vi "VP_NanoPositioner_FPGA_diagonal.vi"() -> ()   [LabVIEW 2015]
uses:
  FPGA states.ctl
  FPGA Commands.ctl
  <vilib>/Platform/TimedLoop/XDataNode/timing_clust.ctl
  <vilib>/Platform/TimedLoop/XDataNode/nitl_modes.ctl
  <vilib>/Platform/TimedLoop/XDataNode/wakeup.ctl
  Control X Up Down Ramp.ctl
  Control Y Up Down Ramp.ctl
  Detector_Trigger_Control.ctl
  <vilib>/rvi/Emulation/niFpgaGetClockAttributes.vi
  <vilib>/rvi/Emulation/niFpgaSctlEmulationGetInTimedLoop.vi
  <vilib>/rvi/Emulation/niFpgaEmulationReportErrorSimple.vi
  <vilib>/rvi/eio/common/nirviEmuTemplateMethod_errors.vi
  <vilib>/rvi/Emulation/niFpgaCriticalErrorInLSC.vi
  <vilib>/rvi/Emulation/niFpgaProcessEmulError.vi
  <vilib>/rvi/interface/RandomDataEmulation/niFpgaRandomDataHandleErrors.vi
  <vilib>/eio/EIONode/EIONode.xnode
  <vilib>/Platform/TimedLoop/XDataNode/XDataNode.xnode
  <vilib>/rvi/DataTransferAndStorage/Container/XNode/niFpgaContainer.xnode
  <vilib>/rvi/interface/RandomDataEmulation/nirviRandomDataFpgaReadWriteTemplate.vi
  <vilib>/rvi/Analysis/measure/butterworth/XNode/niFpgaButterworthFilter.xnode
  <vilib>/Platform/TimedLoop/XDataNode/XDNodeRunTimeDep.lvlib
panel:
  out "Interferometer Loop Error":errorcluster
  out "Fly scan completed":bool
  out "Y scan done":bool=TRUE
  out "X scan done":bool=TRUE
  out "Wait error":errorcluster
  out "Shutdown error":errorcluster
  out "FPGA error monitor":errorcluster
  out "Run Loop error":errorcluster
  in  "Wait timer (ms)":u16=50 caption="Count(mSec)"
  in  "New FPGA command":bool
  in  "FPGA command":T1
  out "FPGA state":T2
  out "End Run Error":errorcluster
  out "Number of Data Strings 2":i32
  out "Measured Data Trigger Time Period (Ticks)":u32
  in  "Data Trigger Time Period (uSec)":u32 caption="Detector Trigger Time Period (uSec)"
  out "Trigger for Data":fxp<+/-,58,25>
  out "Fly Scan Running":bool
  in  "Fly Scan":bool
  out "If True End Y Down Ramp":bool
  in  "Y Ramp Drop Size (nm)":fxp<+/-,16,16>
  out "Ramp Mid Range":bool
  out "If True End Up Ramp":bool
  out "Start or middle":bool=TRUE
  in  "Y Start Marker (nm)":fxp<+/-,58,25> format="%#_55g"
  out "Y Ramp Slope":fxp<+,48,16>
  in  "Y Ramp End (nm)":fxp<+/-,16,16>
  in  "Y Ramp Start (nm)":fxp<+/-,16,16>
  in  "Y Ramp Period (usec)":fxp<+,32,32>
  in  "X Ramp Period (usec)":fxp<+,32,32>
  in  "X Ramp End (nm)":fxp<+/-,16,16>
  in  "X Ramp Start (nm)":fxp<+/-,16,16>
  out "If True End X Down Ramp":bool
  out "X Ramp Mid Range":bool
  out "If True End X Up Ramp":bool
  out "Y Ramp Drop":bool
  out "Next Do Down Ramp":bool
  out "Continue Run":bool
  in  "X Start Marker (nm)":fxp<+/-,58,25>
  out "X Ramp Slope":fxp<+,48,16> format="%.37g"
  in  "DT Reset":bool
  in  "DT Duty Cycle (periods)":fxp<+,32,0>=0.5 caption="DT duty cycle (periods)"
  in  "DT Reference DC Offset (V)":fxp<+/-,16,16>
  in  "DT Reference Amplitude (V)":fxp<+/-,40,17>
  in  "DT Phase Offset (periods)":fxp<+,32,0>
  in  "DT Frequency (periods/tick)":fxp<+,32,0>=0.0002500000409781933
  in  "Trigger Wave Generator":T3(ring)
  out "If True End Trigger Low":bool
  in  "Trigger Low Level (V)":fxp<+/-,20,5>=-5.0
  in  "Trigger High Level (V)":fxp<+/-,20,5>=5.0
  out "If True End Trigger High":bool
  out "Trigger Mid High":bool
  in  "Trigger Low Period (usec)":fxp<+/-,64,45>
  in  "Trigger High Period (usec)":fxp<+/-,64,45>
  out "Measured Z Reference Time Period (Ticks)":u32
  in  "Z Reference Time Period (uSec)":u32
  in  "Z White Noise Amplitude":u16=32767
  in  "Z White Noise Seed":u32=4
  in  "Z Phase Offset (periods)":fxp<+,32,0>
  in  "Z Frequency (periods/tick)":fxp<+,32,0>=0.0002500000409781933
  in  "Z Reference DC Offset (nm)":fxp<+/-,16,16>
  in  "Z Reference Amplitude (nm)":fxp<+/-,40,17>
  in  "Z Reference Reset":bool
  in  "Z Reference Wave Selection":T4(ring)
  in  "Y White Noise Amplitude":u16=32767
  in  "Y White Noise Seed":u32=4
  out "Measured Y Reference Time Period (Ticks)":u32
  in  "Y Reference Time Period (uSec)":u32
  in  "Y Reference Reset":bool
  in  "Y Reference Wave Selection":T5(ring)
  in  "Detector Trigger Lower Limit (V)":fxp<+/-,20,5>=-5.0
  out "Detector Trigger In Range?":bool
  in  "Detector Trigger Upper Limit (V)":fxp<+/-,20,5>=5.0
  out "Detector Trigger (V)":fxp<+/-,20,5> format="%.29g"
  out "Measured Detector Trigger Time Period (Ticks)":u32
  in  "Detector Trigger Time Period (uSec)":u32
  out "Measured Trigger Gen Time Period (Ticks)":u32
  in  "Trigger Generation Time Period (uSec)":u32
  in  "Reference Signal Source":T6(ring)
  in  "Z-Stage Scaling Direction":fxp<+/-,3,3>=-1.0
  in  "Y-Stage Scaling Direction":fxp<+/-,3,3>=-1.0
  in  "Y Phase Offset (periods)":fxp<+,32,0>
  in  "Y Frequency (periods/tick)":fxp<+,32,0>=0.0002500000409781933
  in  "Optics and or Sample Stage":T7(ring)
  out "Z Stage External Reference (nm)":fxp<+/-,58,25>
  in  "Mod 3 AI2 V to nm Scaling":fxp<+,47,18>
  out "Mod 8 Input AI2 (V)":fxp<+/-,24,5>
  out "Y Stage External Reference (nm)":fxp<+/-,58,25>
  in  "Mod 3 AI1 V to nm Scaling":fxp<+,47,18>
  out "Mod 8 Input AI1 (V)":fxp<+/-,24,5>
  in  "Sample Z Stage Resolution (nm)":fxp<+,33,3>=0.001000046730041504
  in  "Sample Y Stage Resolution (nm)":fxp<+,33,3>=0.001000046730041504
  in  "Sample X Stage Resolution (nm)":fxp<+,33,3>=0.001000046730041504
  out "Sample Z Stage Displacement (nm)":fxp<+/-,58,25>
  out "Sample Z Stage Displacement raw (nm)":fxp<+/-,64,35> format="%.62g"
  out "Sample Y Stage Displacement (nm)":fxp<+/-,58,25>
  out "Sample Y Stage Displacement raw (nm)":fxp<+/-,64,35> format="%.41g"
  out "Sample X Stage Displacement raw (nm)":fxp<+/-,64,35> format="%.62g"
  out "Sample X Stage Displacement (nm)":fxp<+/-,58,25>
  in  "Reset Sample Z":bool
  out "32 bit Count Sample  Z":i32
  in  "Reset Sample Y":bool
  out "32 bit Count Sample  Y":i32
  in  "Reset Sample X":bool
  out "32 bit Count Sample X":i32
  out "Mod6/DIO3":bool
  out "Mod6/DIO2":bool
  out "Mod5/DIO3":bool
  out "Mod5/DIO2":bool
  out "Mod4/DIO3":bool
  out "Mod4/DIO2":bool
  out "Measured Analog Input Time Period (Ticks)":u32
  in  "Analog Input Time Period (uSec)":u32
  out "X Stage External Reference (nm)":fxp<+/-,58,25>
  in  "Mod 3 AI0 V to nm Scaling":fxp<+,47,18>
  out "Mod 3 Input AI0 (V)":fxp<+/-,24,5>
  in  "X-Stage Scaling Direction":fxp<+/-,3,3>=-1.0
  in  "Z-Stage nm to V Scaling":fxp<+/-,32,12>
  in  "Y-Stage nm to V Scaling":fxp<+/-,32,12>
  in  "X-Stage nm to V Scaling":fxp<+/-,32,12>
  out "Kxx Output, Kxx*ex (V)":fxp<+/-,58,25>
  out "Kyy Output, Kyy*ey (V)":fxp<+/-,58,25>
  out "Kzz Output, Kzz*ez (V)":fxp<+/-,58,25>
  in  "sos gain SF Controller xx1":fxp<+/-,42,9>
  in  "-a01(2) xx1":fxp<+/-,64,9>[](array[numeric])=[0.0, 0.0, 0.0, 0.0, 0.0, 0.0, 0.0, 0.0, 0.0, 0.0, 0.0, 0.0, 0.0, 0.0, 0.0, 0.0, 0.0, 0.0, 0.0, 0.0]
  in  "-a02(2) xx1":fxp<+/-,64,9>[](array[numeric])=[0.0, 0.0, 0.0, 0.0, 0.0, 0.0, 0.0, 0.0, 0.0, 0.0, 0.0, 0.0, 0.0, 0.0, 0.0, 0.0, 0.0, 0.0, 0.0, 0.0]
  in  "b01(2) xx1":fxp<+/-,64,9>[](array[numeric])=[0.0, 0.0, 0.0, 0.0, 0.0, 0.0, 0.0, 0.0, 0.0, 0.0, 0.0, 0.0, 0.0, 0.0, 0.0, 0.0, 0.0, 0.0, 0.0, 0.0]
  in  "b02(2) xx1":fxp<+/-,64,9>[](array[numeric])=[0.0, 0.0, 0.0, 0.0, 0.0, 0.0, 0.0, 0.0, 0.0, 0.0, 0.0, 0.0, 0.0, 0.0, 0.0, 0.0, 0.0, 0.0, 0.0, 0.0]
  in  "sos gain SF Controller yy1":fxp<+/-,42,9>
  in  "-a01(2) yy1":fxp<+/-,64,9>[](array[numeric])=[0.0, 0.0, 0.0, 0.0, 0.0, 0.0, 0.0, 0.0, 0.0, 0.0, 0.0, 0.0, 0.0, 0.0, 0.0, 0.0, 0.0, 0.0, 0.0, 0.0]
  in  "-a02(2) yy1":fxp<+/-,64,9>[](array[numeric])=[0.0, 0.0, 0.0, 0.0, 0.0, 0.0, 0.0, 0.0, 0.0, 0.0, 0.0, 0.0, 0.0, 0.0, 0.0, 0.0, 0.0, 0.0, 0.0, 0.0]
  in  "b01(2) yy1":fxp<+/-,64,9>[](array[numeric])=[0.0, 0.0, 0.0, 0.0, 0.0, 0.0, 0.0, 0.0, 0.0, 0.0, 0.0, 0.0, 0.0, 0.0, 0.0, 0.0, 0.0, 0.0, 0.0, 0.0]
  in  "b02(2) yy1":fxp<+/-,64,9>[](array[numeric])=[0.0, 0.0, 0.0, 0.0, 0.0, 0.0, 0.0, 0.0, 0.0, 0.0, 0.0, 0.0, 0.0, 0.0, 0.0, 0.0, 0.0, 0.0, 0.0, 0.0]
  in  "sos gain SF Controller zz1":fxp<+/-,42,9>
  in  "-a01(2) zz1":fxp<+/-,64,9>[](array[numeric])=[0.0, 0.0, 0.0, 0.0, 0.0, 0.0, 0.0, 0.0, 0.0, 0.0, 0.0, 0.0, 0.0, 0.0, 0.0, 0.0, 0.0, 0.0, 0.0, 0.0]
  in  "-a02(2) zz1":fxp<+/-,64,9>[](array[numeric])=[0.0, 0.0, 0.0, 0.0, 0.0, 0.0, 0.0, 0.0, 0.0, 0.0, 0.0, 0.0, 0.0, 0.0, 0.0, 0.0, 0.0, 0.0, 0.0, 0.0]
  in  "b01(2) zz1":fxp<+/-,64,9>[](array[numeric])=[0.0, 0.0, 0.0, 0.0, 0.0, 0.0, 0.0, 0.0, 0.0, 0.0, 0.0, 0.0, 0.0, 0.0, 0.0, 0.0, 0.0, 0.0, 0.0, 0.0]
  in  "b02(2) zz1":fxp<+/-,64,9>[](array[numeric])=[0.0, 0.0, 0.0, 0.0, 0.0, 0.0, 0.0, 0.0, 0.0, 0.0, 0.0, 0.0, 0.0, 0.0, 0.0, 0.0, 0.0, 0.0, 0.0, 0.0]
  in  "Scaling mV to V":fxp<+,33,10>=0.0009765625
  in  "System Loop Type":enum16{"Open Loop", "Closed Loop"}(ring)
  in  "Timeout FPGA FIFO1":i32=40000000
  out "FIFO Timed Out":bool
  out "Number of Data Strings":i32
  in  "Y Reference DC Offset (nm)":fxp<+/-,16,16>
  in  "X Reference DC Offset (nm)":fxp<+/-,16,16>
  in  "Y Reference Amplitude (nm)":fxp<+/-,40,17>
  out "Z Stage Reference (nm)":fxp<+/-,58,25> format="%.41g"
  out "Y Stage Reference (nm)":fxp<+/-,58,25> format="%.41g"
  out "Optics Z Stage Displacement (nm)":fxp<+/-,58,25>
  out "Optics Z Stage Displacement raw (nm)":fxp<+/-,64,35>
  in  "Optics Z Stage Resolution (nm)":fxp<+,33,3>=0.001000046730041504
  in  "Reset Optics Z":bool
  out "32 bit Count Optics  Z":i32
  out "Mod6/DIO1":bool
  out "Mod6/DIO0":bool
  out "Optics Y Stage Displacement (nm)":fxp<+/-,58,25>
  out "Optics Y Stage Displacement raw (nm)":fxp<+/-,64,35>
  in  "Optics Y Stage Resolution (nm)":fxp<+,33,3>=0.001000046730041504
  in  "Reset Optics Y":bool
  out "32 bit Count Optics  Y":i32
  out "Mod5/DIO1":bool
  out "Mod5/DIO0":bool
  out "Z-Stage Input In Range?":bool
  out "Y-Stage Input In Range?":bool
  in  "Controller Output Lower Limit":fxp<+/-,20,5>=-5.0
  out "X-Stage Input In Range?":bool
  in  "Controller Output Upper Limit":fxp<+/-,20,5>=5.0
  in  "X White Noise Amplitude":u16=32767
  in  "X White Noise Seed":u32=4
  in  "X Reference Reset":bool
  in  "X Reference Wave Selection":T8(ring)
  out "Measured Counter Time Period (Ticks)":u32
  out "Measured Datalog Time Period (Ticks)":u32
  out "Measured Plant Output Time Period (Ticks)":u32
  out "Measured Controller Output Time Period (Ticks)":u32
  out "Measured Controller Time Period (Ticks)":u32
  out "Measured X Reference Time Period (Ticks)":u32
  out "Optics X Stage Displacement raw (nm)":fxp<+/-,64,35>
  in  "Optics X Stage Resolution (nm)":fxp<+,33,3>=0.001000046730041504 format="%#_31g"
  in  "Plant Output Time Period (uSec)":u32
  out "Optics X Stage Displacement (nm)":fxp<+/-,58,25>
  in  "Reset Optics X":bool
  out "32 bit Count Optics X":i32
  out "Mod4/DIO1":bool
  out "Mod4/DIO0":bool
  out "Start Run Error":errorcluster
  out "stop case":bool
  in  "Controller Output Time Period (uSec)":u32
  in  "Datalog Cases":T9(ring)
  out "PI Z-Stage Input (V)":fxp<+/-,20,5> format="%.29g"
  out "PI Y-Stage Input (V)":fxp<+/-,20,5> format="%.29g"
  out "PI X-Stage Input (V)":fxp<+/-,20,5> format="%.29g"
  in  "Controller Time Period (uSec)":u32
  in  "Datalog Time Period (uSec)":u32
  in  "X Reference Time Period (uSec)":u32
  in  "X Reference Amplitude (nm)":fxp<+/-,40,17>
  out "X Stage Reference (nm)":fxp<+/-,58,25> format="%.41g"
  out "FIFO Timed Out?":bool
  in  "X Phase Offset (periods)":fxp<+,32,0>
  in  "X Frequency (periods/tick)":fxp<+,32,0>=0.0002500000409781933
types:
  T1 = typedef "FPGA Commands.ctl" = enum16{"Start Scan", "Shutdown"}
  T2 = typedef "FPGA states.ctl" = enum16{"Wait", "Start Run", "Run", "End Run", "Shutdown"}
  T3 = enum16{"Custom Square Wave ", "Square Wave 1", "Square Wave 2"}
  T4 = enum16{"Constant", "Sine Wave", "Sawtooth Wave", "Square Wave", "Filtered White Noise"}
  T5 = enum16{"Constant", "Sine Wave", "Custom Ramp Wave", "Filtered White Noise"}
  T6 = enum16{"FPGA Generated Reference", "External Reference"}
  T7 = enum16{"Optics Stage Only", "Optics and Sample Stage"}
  T8 = enum16{"Constant", "Sine Wave", "Custom Up Down Ramp", "Filtered White Noise"}
  T9 = enum16{"Data Log 1", "Data Log 2", "Data Log 3", "Data Log 4", "Data Log 5", "Data Log 6", "Data Log 7", "Data Log 8", "Data Log 9", "Data Log 10", "Data Log 11", "Data Log 12", "Data Log 13", "Data Log 14", "Data Log 15", "Data Log 16"}
  T10 = typedef "Control Y Up Down Ramp.ctl" = enum16{"Y Up Ramp", "Y Down Ramp"}
  T11 = typedef "Detector_Trigger_Control.ctl" = enum16{"Trigger High", "Trigger Low"}
  T12 = typedef "Control X Up Down Ramp.ctl" = enum16{"X Up Ramp", "X Down Ramp"}
  T13 = typedef "XDNodeRunTimeDep.lvlib/timing_clust.ctl" = cluster{"Expected End [f-1]":u64, "Actual End [f-1]":u64, "Finished Late? [f-1]":bool, "Expected End [i-1]":u64, "Actual End [i-1]":u64, "Finished Late? [i-1]":bool, "Expected Start [i]":u64, "Actual Start [i]":u64, "Expected Start [f]":u64, "Actual Start [f]":u64, "Source Name":string, "Structure Name":string, "Period":i64, "Deadline":i64, "Offset":i64, "Start":i64, "Priority":i32, "Timeout":i32, "Mode":T14, "Wakeup Reason":T15, "Error":errorcluster, "Source Type":string, "Secondary Source Type":string, "Global End Time":u64, "Global Start Time":u64, "Frame Duration":u64, "Iteration Duration":u64, "Assigned CPU":i32, "I/O Scan Engine Mode":u32}
  T14 = typedef "XDNodeRunTimeDep.lvlib/nitl_modes.ctl" = enum32{"No Change", "Process missed periods, maintain original phase", "Discard missed periods, maintain original phase", "Process missed periods, ignore original phase", "Discard missed periods, ignore original phase"}
  T15 = typedef "XDNodeRunTimeDep.lvlib/wakeup.ctl" = enum32{"Normal", "Aborted", "Asynchronous wakeup", "Timing source error", "Timed loop error", "Timeout"}
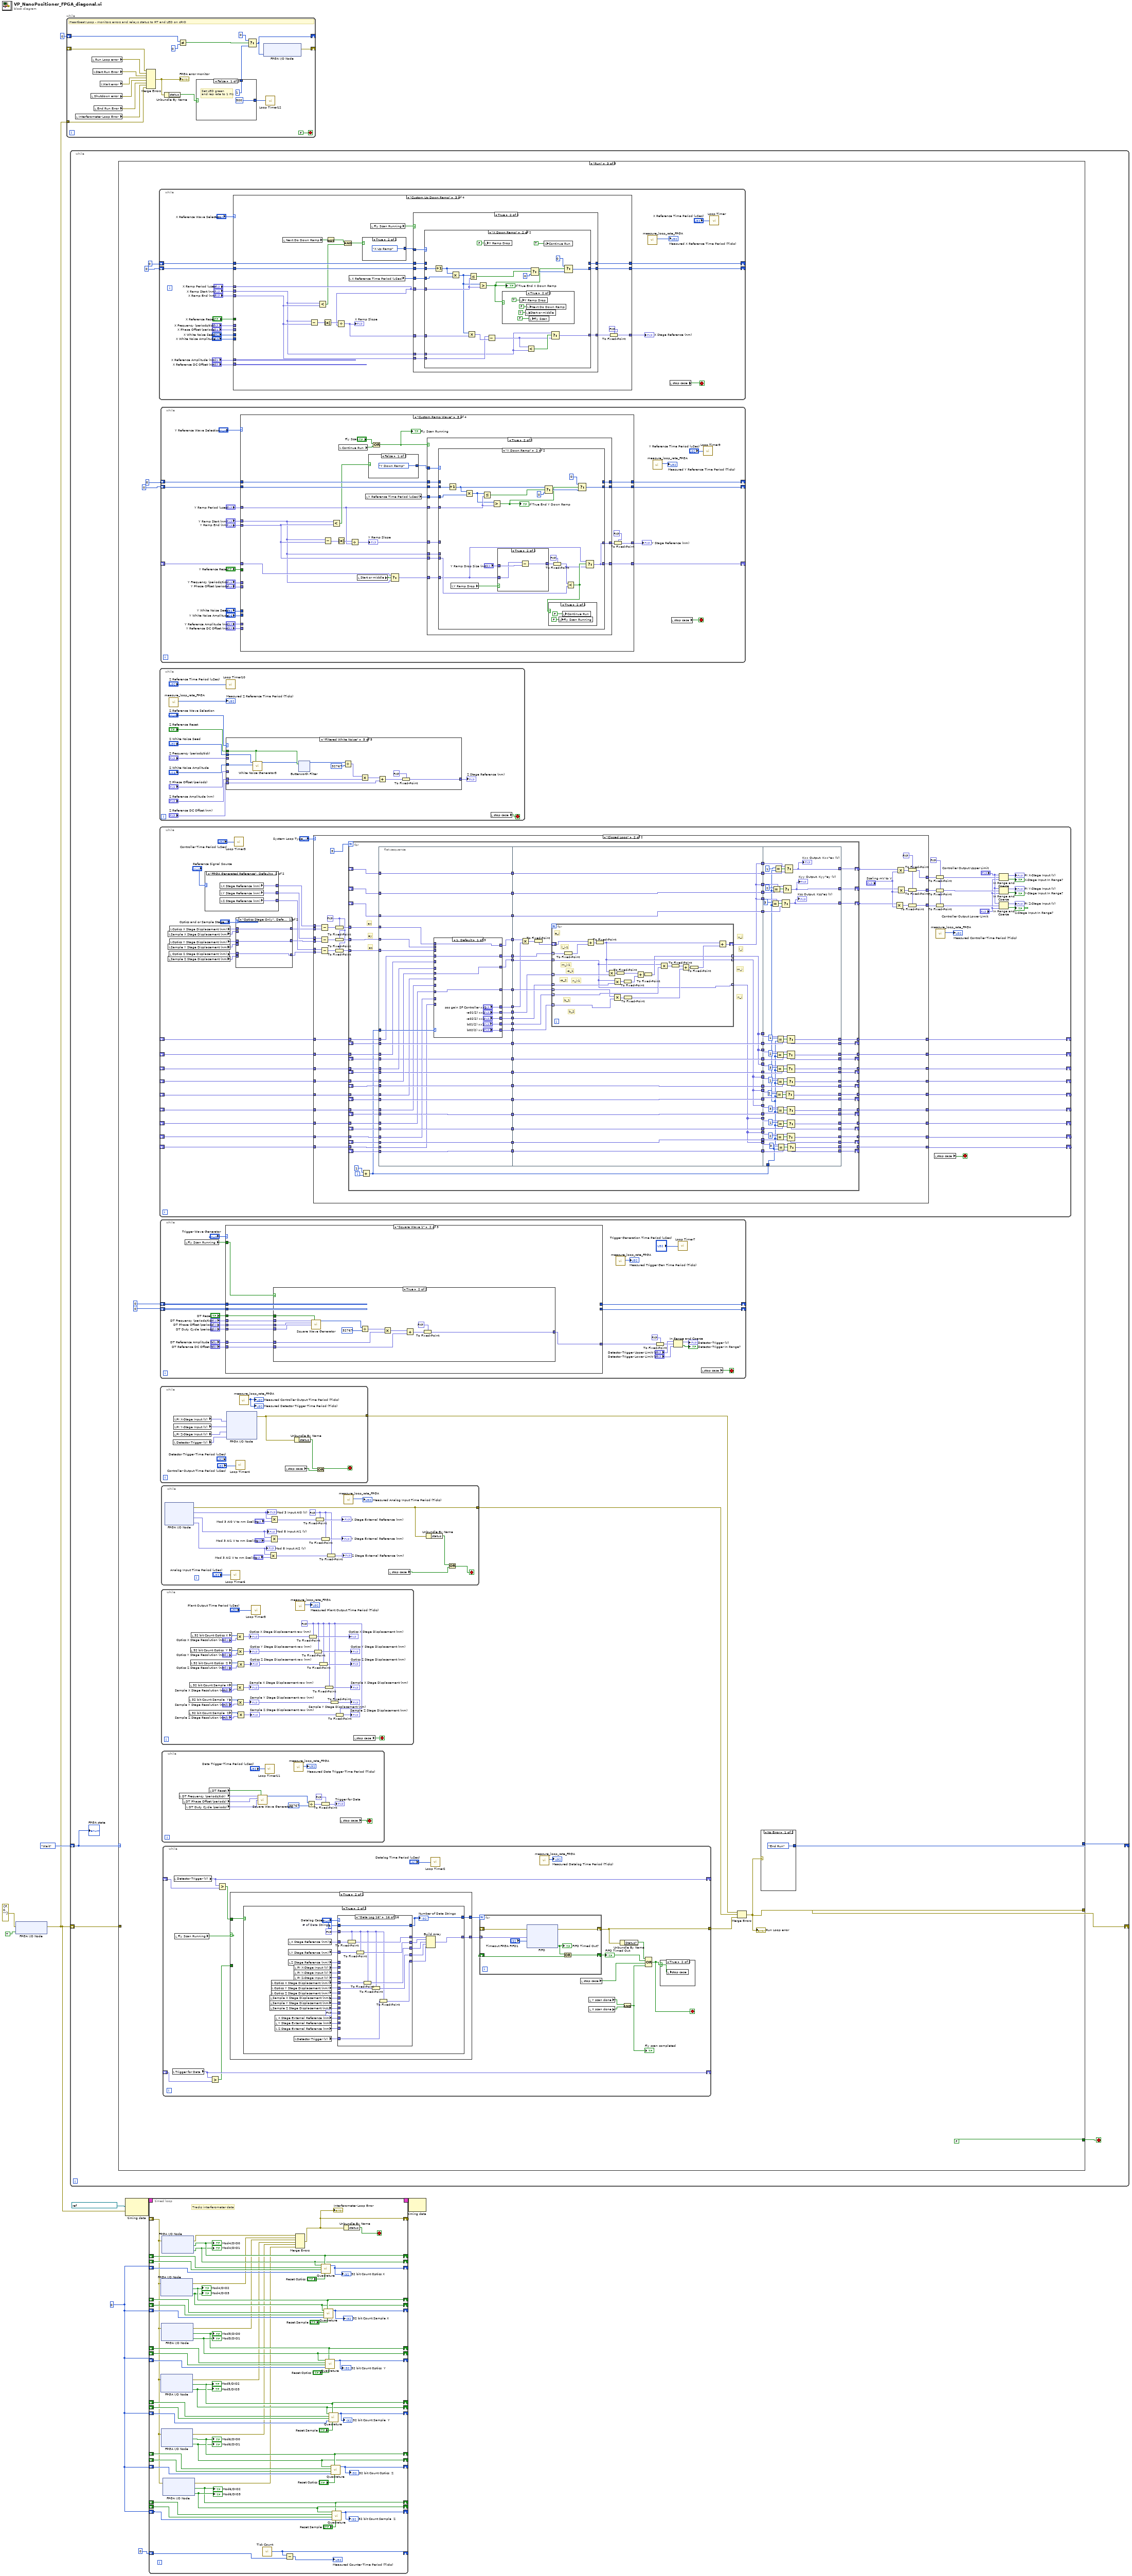
[diagram p0: block diagram]
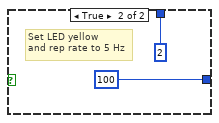
[diagram p2: hidden frame]
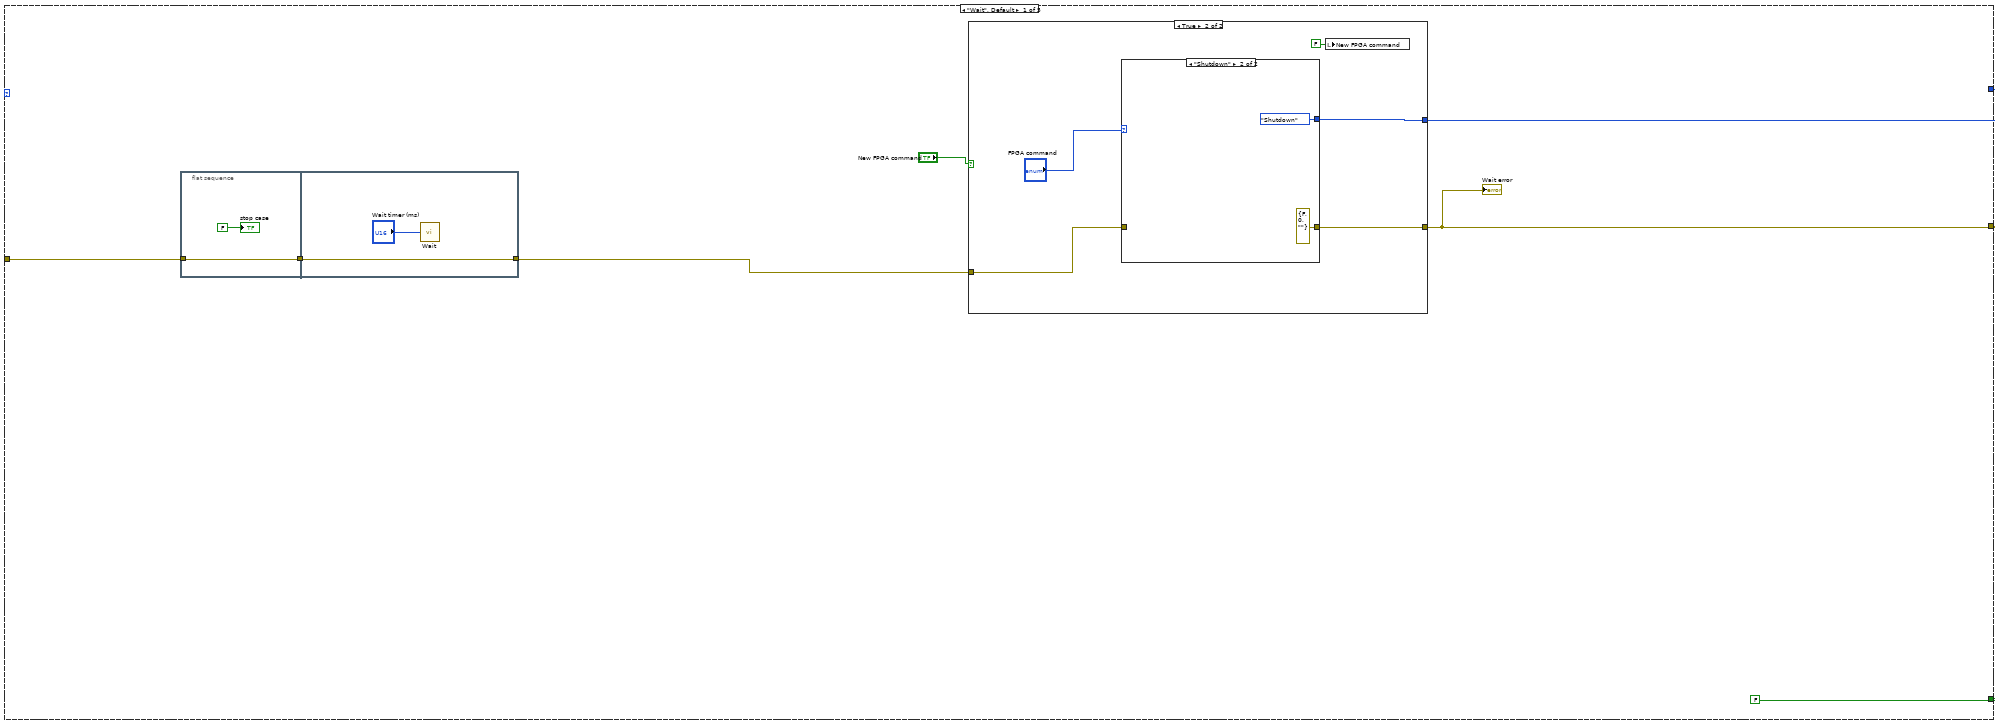
[diagram p3: hidden frame]
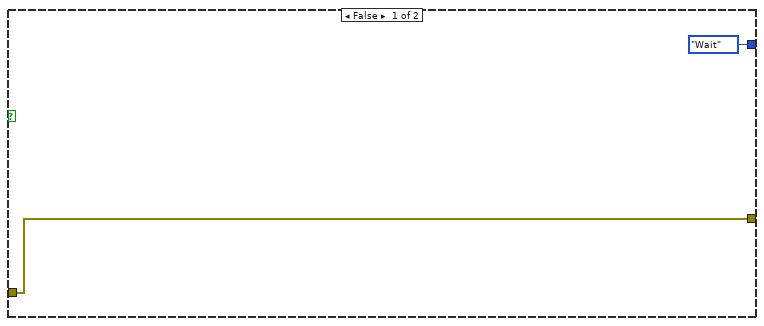
[diagram p4: hidden frame]
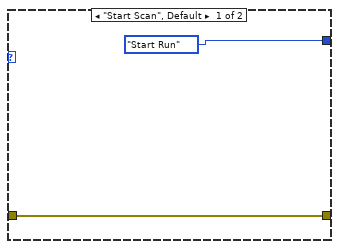
[diagram p5: hidden frame]
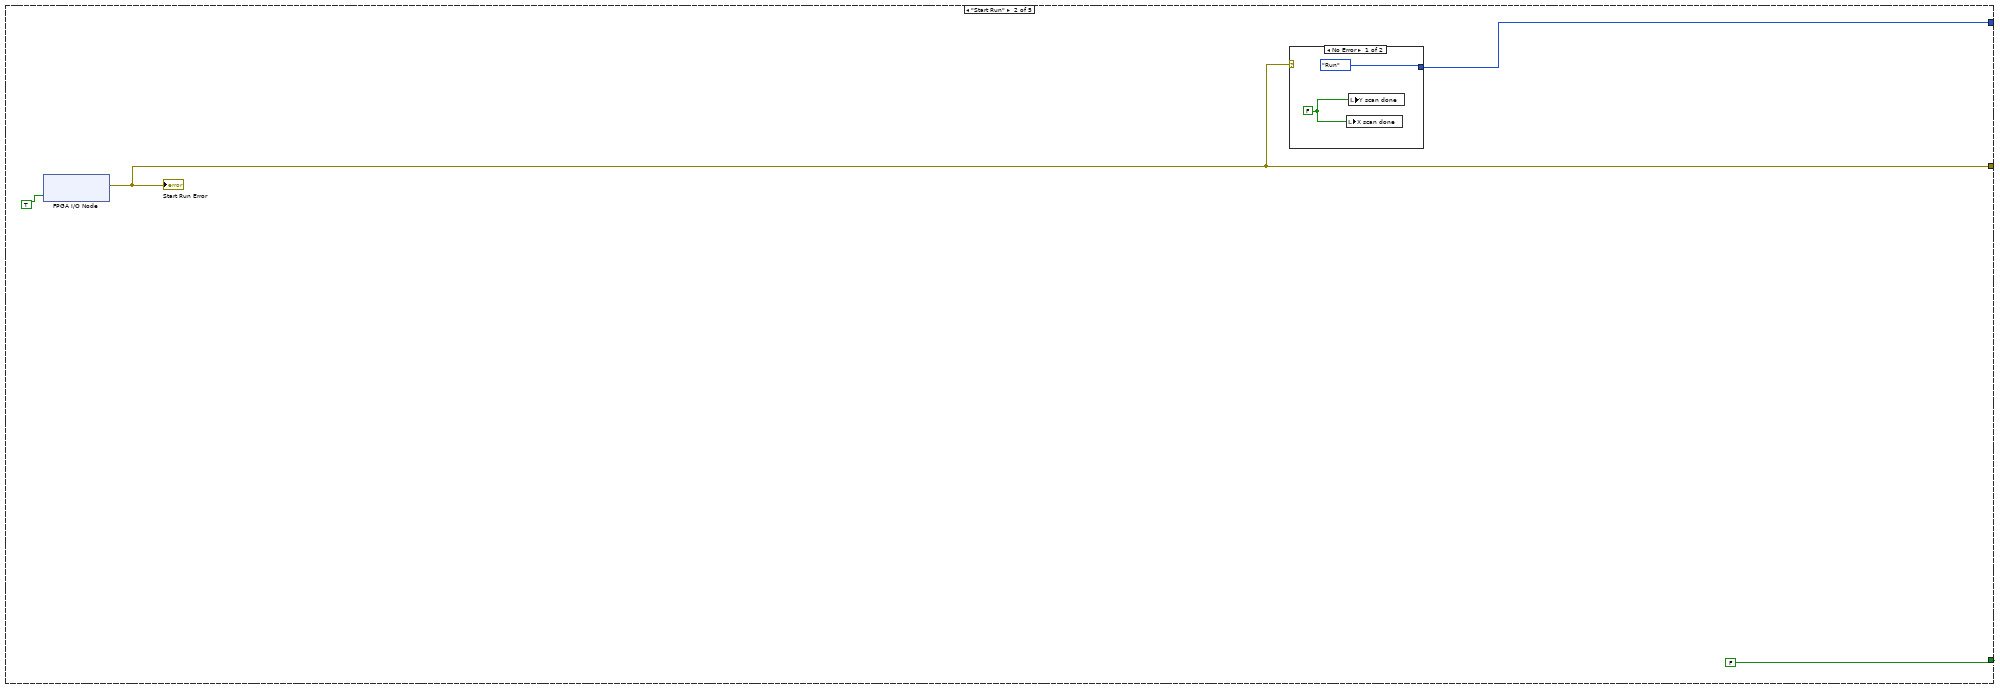
[diagram p6: hidden frame]
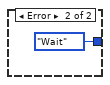
[diagram p7: hidden frame]
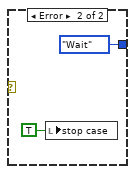
[diagram p8: hidden frame]
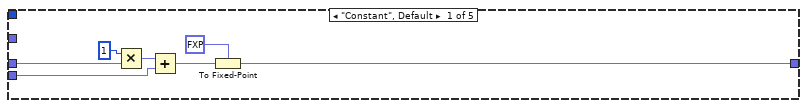
[diagram p9: hidden frame]
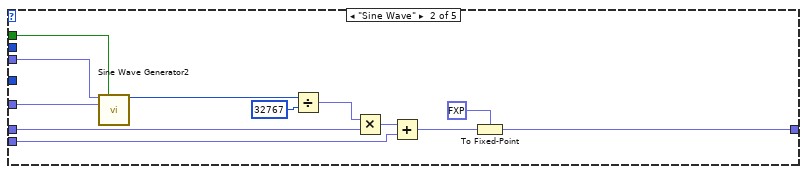
[diagram p10: hidden frame]
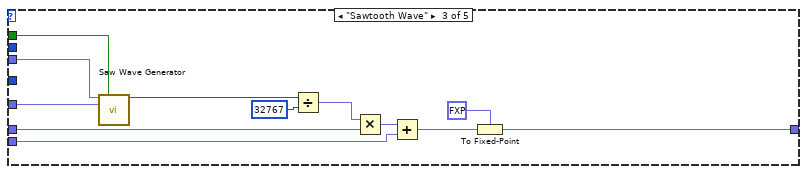
[diagram p11: hidden frame]
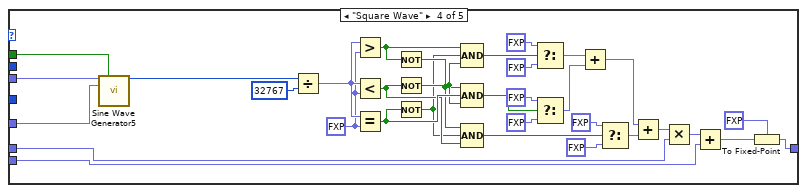
[diagram p12: hidden frame]
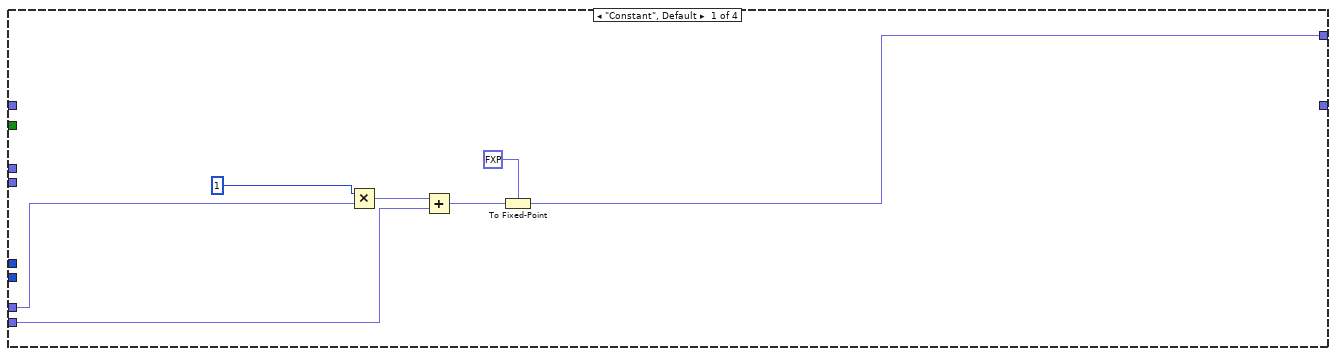
[diagram p13: hidden frame]
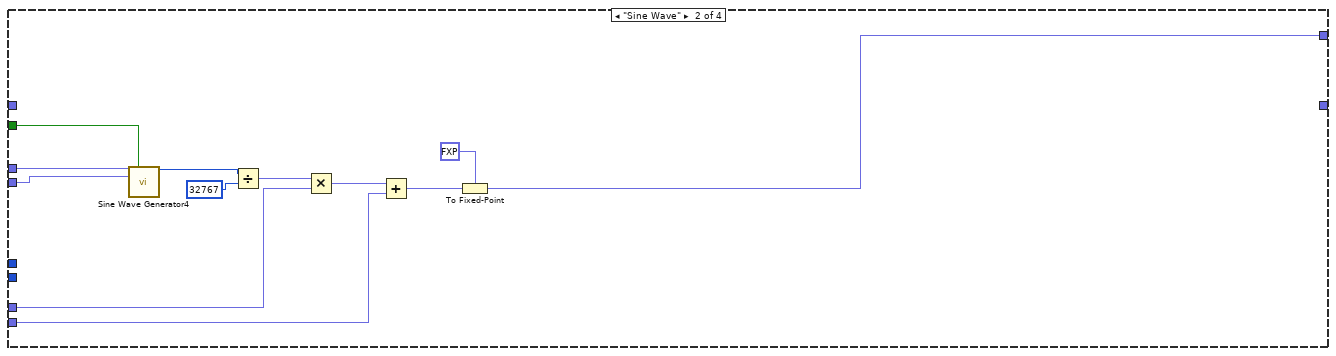
[diagram p14: hidden frame]
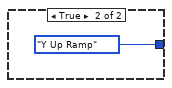
[diagram p15: hidden frame]
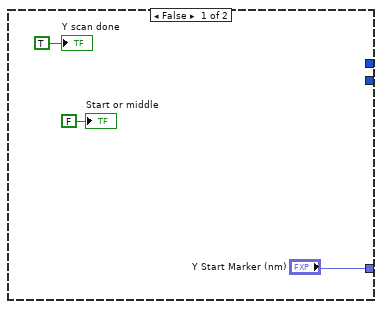
[diagram p16: hidden frame]
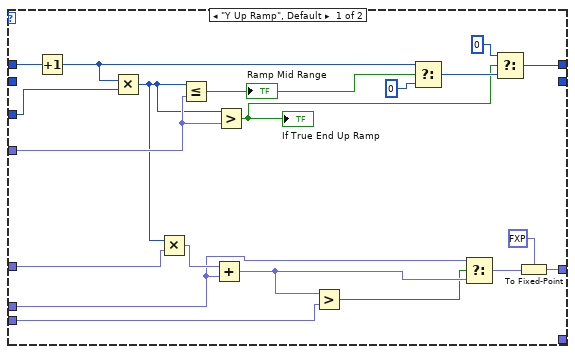
[diagram p17: hidden frame]
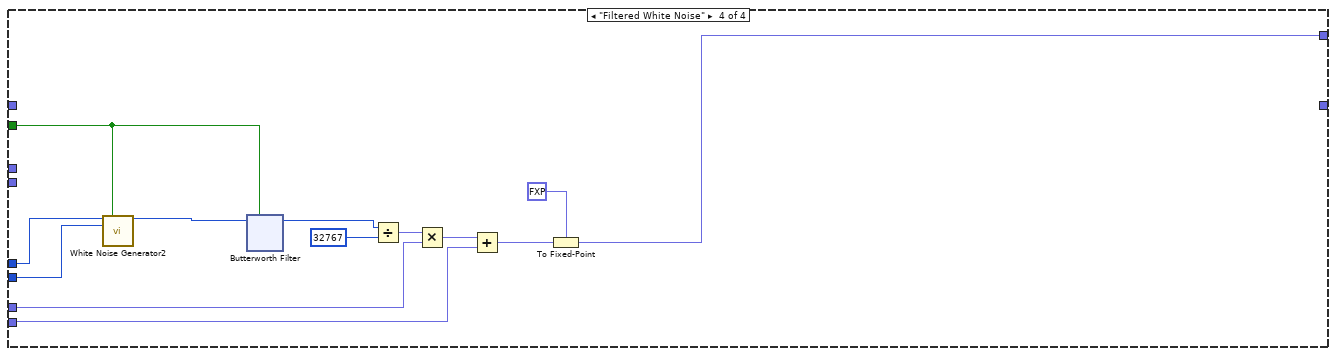
[diagram p20: hidden frame]
diagram:
  w4 = 0 ("Tick Count(Ticks)")
  n1 = xnode "FPGA I/O Node"("error in"=errorcluster {"status"=FALSE, "code"=0, "source"=""} ("error IO"), "Mod3/Start"=TRUE ("I/O Item")) -> ("error out"=w1:errorcluster)  [unwired: 1 in, 1 out]
  n2 = while {
    tunnel: w1 -> [w24]
    shift-right: [w22] -> _
    shift-left: _ -> [w21]
    shift-right: [w19] -> _
    shift-left: u8 0 ("USER FPGA LED") -> [w17]
    stop <- FALSE stop-if-true
    # "Heartbeat Loop - monitors errors and relays status to RT and LED on cRIO"
    n3 = local read "Interferometer Loop Error"() -> (w11:errorcluster)
    n4 = local read "Shutdown error"() -> (w26:errorcluster)
    n5 = local read "Run Loop error"() -> (w29:errorcluster)
    n6 = local read "Start Run Error"() -> (w28:errorcluster)
    n7 = local read "End Run Error"() -> (w25:errorcluster)
    n8 = local read "Wait error"() -> (w27:errorcluster)
    n9 = Merge Errors(w21, w29, w28, w27, w26, w25, w11, w24) -> (w23:errorcluster)
    "FPGA error monitor" <- w23
    n10 = Unbundle By Name(w23) -> ("status"=w12:bool)
    n11 = Not Equal?(x=w17, y=u8 0) -> (x != y?=w15:bool)
    n12 = case shown="False" w12 {
      tunnel: [u16 500 ("Count(mSec)") u16 100 ("Count(mSec)")] -> w20
      tunnel: [u8 1 ("USER FPGA LED") u8 2 ("USER FPGA LED")] -> w13
      frame False {
        # "Set LED green \nand rep rate to 1 Hz"
      }
      frame True {
        # "Set LED yellow \nand rep rate to 5 Hz"
      }
    }
    n13 = Select(t=u8 0, s=w15, f=w13) -> (s? t:f=w19:u8)
    n14 = xnode "FPGA I/O Node"("USER FPGA LED"=w19) -> ("error out"=w22:errorcluster)  [unwired: 2 in, 1 out]
    n15 = call "Loop Timer12"("Count(mSec)"=w20) -> ()  [unwired: 1 out]
  }
  n16 = while {
    shift-right: [w36] -> _
    shift-left: FPGA_states."Wait" -> [w38]
    shift-right: [w35] -> _
    shift-left: w1 -> [w34]
    stop <- w37 stop-if-true
    n17 = case shown="\"Run\"" w38 {
      tunnel: [w43 w61 w69 w1343 w1347] -> w35
      tunnel: [FALSE FALSE FALSE FALSE TRUE] -> w37
      tunnel: [w45 w62 w70 FPGA_states."Wait" FPGA_states."Shutdown"] -> w36
      tunnel: w34 -> [w40 _ _ _ w1348]
      frame "Wait", Default {
        n18 = flat-sequence {
          tunnel: w40 -> [w46]
          tunnel: [w46] -> w41
          tunnel: [w48] -> w39
          tunnel: w41 -> [w48]
          frame #0 {
            "stop case" <- FALSE ("stop case")
          }
          frame #1 {
            n19 = call "Wait"("Count(mSec)"="Wait timer (ms)") -> ()  [unwired: 1 out]
          }
        }
        n20 = case shown="True" "New FPGA command" {
          tunnel: [FPGA_states."Wait" w56] -> w45
          tunnel: w39 -> [w51 w55]
          tunnel: [w51 w54] -> w43
          frame False {
          }
          frame True {
            n21 = case shown="\"Shutdown\"" "FPGA command" {
              tunnel: [FPGA_states."Start Run" FPGA_states."Shutdown"] -> w56
              tunnel: w55 -> [w57 _]
              tunnel: [w57 errorcluster {"status"=FALSE, "code"=0, "source"=""} ("error IO")] -> w54
              frame "Start Scan", Default {
              }
              frame "Shutdown" {
              }
            }
            n22 = local write "New FPGA command"(FALSE ("New FPGA command")) -> ()
          }
        }
        "Wait error" <- w43
      }
      frame "Start Run" {
        n23 = xnode "FPGA I/O Node"("Mod3/Start"=TRUE ("I/O Item")) -> ("error out"=w61:errorcluster)  [unwired: 2 in, 1 out]
        "Start Run Error" <- w61
        n24 = case shown="No Error" w61 {
          tunnel: [FPGA_states."Run" FPGA_states."Wait"] -> w62
          frame No Error {
            w65 = FALSE
            n25 = local write "X scan done"(w65) -> ()
            n26 = local write "Y scan done"(w65) -> ()
          }
          frame Error {
          }
        }
      }
      frame "Run" {
        n27 = while {
          shift-right: [w1204] -> _
          shift-left: u32 0 ("f") -> [w1202]
          shift-right: [w1203] -> _
          shift-left: u32 0 -> [w1201]
          stop <- w1213 stop-if-true
          n28 = case shown="\"Custom Up Down Ramp\"" "X Reference Wave Selection" {
            tunnel: "X Frequency (periods/tick)" -> [_ w1235 _ _]
            tunnel: "X Phase Offset (periods)" -> [_ w1234 _ _]
            tunnel: "X Reference Reset" -> [_ w1232 _ w1331]
            tunnel: "X White Noise Seed" -> [_ _ _ w1333]
            tunnel: "X White Noise Amplitude" -> [_ _ _ w1330]
            tunnel: "X Reference Amplitude (nm)" -> [w1220 w1227 _ w1321]
            tunnel: "X Reference DC Offset (nm)" -> [w1219 w1226 _ w1322]
            tunnel: [w1218 w1225 w1239 w1324] -> w1206
            tunnel: [_ _ w1252 _] -> w1204
            tunnel: [_ _ w1251 _] -> w1203
            tunnel: w1202 -> [_ _ w1250 _]
            tunnel: w1201 -> [_ _ w1249 _]
            tunnel: "X Ramp Period (usec)" -> [_ _ w1248 _]
            tunnel: "X Ramp Start (nm)" -> [_ _ w1237 _]
            tunnel: "X Ramp End (nm)" -> [_ _ w1238 _]
            frame "Constant", Default {
              n29 = Multiply(x=i16 1 ("y"), y=w1220) -> (x*y=w1223:fxp<+/-,56,33>)
              n30 = Add(x=w1223, y=w1219) -> (x+y=w1222:fxp<+/-,56,33>)
              n31 = To Fixed-Point(fixed-point type=fxp<+/-,58,25> 0.0, number=w1222) -> (fixed-point=w1218:fxp<+/-,58,25>)
            }
            frame "Sine Wave" {
              n32 = call "Sine Wave Generator"("frequency (periods/tick)"=w1235, "reset"=w1232, "phase offset (periods)"=w1234) -> ("sine out"=w1233:i16)  [unwired: 12 in]
              n33 = Divide(x=w1233, y=i16 32767) -> (x/y=w1228:fxp<+/-,41,18>)
              n34 = Multiply(x=w1228, y=w1227) -> (x*y=w1230:fxp<+/-,64,35>)
              n35 = Add(x=w1230, y=w1226) -> (x+y=w1229:fxp<+/-,64,36>)
              n36 = To Fixed-Point(fixed-point type=fxp<+/-,58,25> 0.0, number=w1229) -> (fixed-point=w1225:fxp<+/-,58,25>)
            }
            frame "Custom Up Down Ramp" {
              n37 = local read "Next Do Down Ramp"() -> (w1244:bool)
              n38 = Subtract(x=w1237, y=w1238) -> (x-y=w1254:fxp<+/-,17,17>)
              n39 = Less?(x=w1237, y=w1238) -> (x < y?=w1243:bool)
              n40 = Absolute Value(x=w1254) -> (abs(x)=w1253:fxp<+,16,16>)
              n41 = Not(x=w1244) -> (.not. x?=w1245:bool)
              n42 = Divide(x=w1253, y=w1248) -> (x/y=w1255:fxp<+,48,16>)
              "X Ramp Slope" <- w1255
              n43 = Compound Arithmetic op=AND(w1245, w1243) -> (w1246:bool)
              n44 = local read "X Reference Time Period (uSec)"() -> (w1247:u32)
              n45 = case shown="True" w1246 {
                tunnel: [Control_X_Up_Down_Ramp."X Down Ramp" Control_X_Up_Down_Ramp."X Up Ramp"] -> w1242
                frame False {
                }
                frame True {
                }
              }
              n46 = local read "Fly Scan Running"() -> (w1241:bool)
              n47 = case shown="True" w1241 {
                tunnel: w1242 -> [_ w1272]
                tunnel: w1247 -> [_ w1271]
                tunnel: ["X Start Marker (nm)" w1270] -> w1240
                tunnel: w1248 -> [_ w1269]
                tunnel: w1255 -> [_ w1268]
                tunnel: w1237 -> [_ w1267]
                tunnel: w1238 -> [_ w1266]
                tunnel: [_ w1265] -> w1252
                tunnel: [_ w1264] -> w1251
                tunnel: w1250 -> [_ w1263]
                tunnel: w1249 -> [_ w1262]
                frame False {
                  n48 = local write "Next Do Down Ramp"(FALSE ("Restart Up Ramp")) -> ()
                  n49 = local write "Y Ramp Drop"(FALSE ("Y Toggle 1")) -> ()
                  "X scan done" <- TRUE
                }
                frame True {
                  n50 = case shown="\"X Down Ramp\"" w1272 {
                    tunnel: [w1291 _] -> w1265
                    tunnel: w1263 -> [w1290 _]
                    tunnel: w1271 -> [w1287 w1312]
                    tunnel: w1269 -> [w1286 w1308]
                    tunnel: w1267 -> [w1277 w1299]
                    tunnel: w1266 -> [w1275 w1300]
                    tunnel: [_ w1315] -> w1264
                    tunnel: w1262 -> [_ w1314]
                    tunnel: w1268 -> [w1282 w1306]
                    tunnel: [w1279 w1302] -> w1270
                    frame "X Up Ramp", Default {
                      n51 = Increment(x=w1290) -> (x+1=w1288:u32)
                      n52 = Multiply(x=w1288, y=w1287) -> (x*y=w1283:u32)
                      n53 = Multiply(x=w1283, y=w1282) -> (x*y=w1281:fxp<+,64,48>)
                      n54 = Less Or Equal?(x=w1283, y=w1286) -> (x <= y?=w1285:bool)
                      "X Ramp Mid Range" <- w1285
                      n55 = Add(x=w1281, y=w1277) -> (x+y=w1280:fxp<+/-,64,50>)
                      n56 = Greater?(x=w1283, y=w1286) -> (0:w1276:bool)
                      "If True End X Up Ramp" <- w1276
                      n57 = local write "Y Ramp Drop"(FALSE ("Y Ramp Drop")) -> ()
                      n58 = case shown="True" w1276 {
                        frame False {
                        }
                        frame True {
                          n59 = local write "Start or middle"(TRUE ("Start or middle")) -> ()
                          n60 = local write "Fly Scan"(FALSE ("Fly Scan Start")) -> ()
                          "Y Ramp Drop" <- TRUE ("Boolean")
                          "Next Do Down Ramp" <- TRUE
                        }
                      }
                      n61 = Greater?(x=w1280, y=w1275) -> (0:w1278:bool)
                      n62 = Select(t=w1288, s=w1285, f=u32 0) -> (s? t:f=w1289:u32)
                      n63 = Select(t=w1275, s=w1278, f=w1280) -> (s? t:f=w1279:fxp<+/-,64,50>)
                      n64 = Select(t=u32 0, s=w1276, f=w1289) -> (s? t:f=w1291:u32)
                      "Continue Run" <- TRUE ("Fly Scan Running")
                    }
                    frame "X Down Ramp" {
                      n65 = Increment(x=w1314) -> (x+1=w1313:u32)
                      n66 = Multiply(x=w1313, y=w1312) -> (x*y=w1307:u32)
                      n67 = Multiply(x=w1307, y=w1306) -> (x*y=w1305:fxp<+,64,48>)
                      n68 = Less Or Equal?(x=w1307, y=w1308) -> (x <= y?=w1311:bool)
                      n69 = Greater?(x=w1307, y=w1308) -> (0:w1301:bool)
                      "If True End X Down Ramp" <- w1301
                      n70 = local write "Y Ramp Drop"(FALSE ("Y Ramp Drop")) -> ()
                      n71 = Subtract(x=w1300, y=w1305) -> (x-y=w1303:fxp<+/-,64,50>)
                      n72 = case shown="True" w1301 {
                        frame False {
                        }
                        frame True {
                          n73 = local write "Y Ramp Drop"(TRUE ("Start Scan")) -> ()
                          n74 = local write "Start or middle"(TRUE ("Start or middle")) -> ()
                          n75 = local write "Next Do Down Ramp"(FALSE ("Next Do Down Ramp")) -> ()
                          n76 = local write "Fly Scan"(FALSE ("Fly Scan Start")) -> ()
                        }
                      }
                      n77 = Less?(x=w1303, y=w1299) -> (x < y?=w1304:bool)
                      n78 = Select(t=w1313, s=w1311, f=u32 0) -> (s? t:f=w1309:u32)
                      n79 = local write "Continue Run"(TRUE ("Fly Scan Running")) -> ()
                      n80 = Select(t=w1299, s=w1304, f=w1303) -> (s? t:f=w1302:fxp<+/-,64,50>)
                      n81 = Select(t=u32 0, s=w1301, f=w1309) -> (s? t:f=w1315:u32)
                    }
                  }
                }
              }
              n82 = To Fixed-Point(fixed-point type=fxp<+/-,58,25> 0.0, number=w1240) -> (fixed-point=w1239:fxp<+/-,58,25>)
            }
            frame "Filtered White Noise" {
              n83 = call "White Noise Generator"("seed"=w1333, "reset"=w1331, "amplitude"=w1330) -> ("white noise out"=w1332:i16)  [unwired: 12 in]
              n84 = xnode "Butterworth Filter"("input data"=w1332, "reset"=w1331) -> ("output data"=w1328:i16)  [unwired: 1 in]
              n85 = Divide(x=w1328, y=i16 32767) -> (x/y=w1323:fxp<+/-,41,18>)
              n86 = Multiply(x=w1323, y=w1321) -> (x*y=w1326:fxp<+/-,64,35>)
              n87 = Add(x=w1326, y=w1322) -> (x+y=w1325:fxp<+/-,64,36>)
              n88 = To Fixed-Point(fixed-point type=fxp<+/-,58,25> 0.0, number=w1325) -> (fixed-point=w1324:fxp<+/-,58,25>)
            }
          }
          "X Stage Reference (nm)" <- w1206
          n89 = call "measure_loop_rate_FPGA.vi"() -> ("Loop Rate (Ticks)"=→"Measured X Reference Time Period (Ticks)":u32)  [unwired: 11 in]
          n90 = local read "stop case"() -> (w1213:bool)
          n91 = call "Loop Timer"("Count(uSec)"="X Reference Time Period (uSec)") -> ()  [unwired: 1 out]
        }
        n92 = while {
          stop <- w95 stop-if-true
          n93 = call "measure_loop_rate_FPGA.vi"() -> ("Loop Rate (Ticks)"=→"Measured Z Reference Time Period (Ticks)":u32)  [unwired: 11 in]
          n94 = call "Loop Timer10"("Count(uSec)"="Z Reference Time Period (uSec)") -> ()  [unwired: 1 out]
          n95 = case shown="\"Filtered White Noise\"" "Z Reference Wave Selection" {
            tunnel: "Z Reference Reset" -> [_ w125 w132 w148 w181]
            tunnel: "Z Frequency (periods/tick)" -> [_ w124 w131 w147 _]
            tunnel: "Z Phase Offset (periods)" -> [_ w123 w130 w146 _]
            tunnel: "Z White Noise Seed" -> [_ _ _ _ w183]
            tunnel: "Z White Noise Amplitude" -> [_ _ _ _ w182]
            tunnel: "Z Reference DC Offset (nm)" -> [w107 w116 w127 w138 w172]
            tunnel: "Z Reference Amplitude (nm)" -> [w108 w117 w126 w140 w173]
            tunnel: [w109 w114 w128 w143 w171] -> w96
            frame "Constant", Default {
              n96 = Multiply(x=i16 1 ("y"), y=w108) -> (x*y=w112:fxp<+/-,56,33>)
              n97 = Add(x=w112, y=w107) -> (x+y=w111:fxp<+/-,56,33>)
              n98 = To Fixed-Point(fixed-point type=fxp<+/-,58,25> 0.0, number=w111) -> (fixed-point=w109:fxp<+/-,58,25>)
            }
            frame "Sine Wave" {
              n99 = call "Sine Wave Generator2"("frequency (periods/tick)"=w124, "reset"=w125, "phase offset (periods)"=w123) -> ("sine out"=w118:i16)  [unwired: 12 in]
              n100 = Divide(x=w118, y=i16 32767) -> (x/y=w121:fxp<+/-,41,18>)
              n101 = Multiply(x=w121, y=w117) -> (x*y=w120:fxp<+/-,64,35>)
              n102 = Add(x=w120, y=w116) -> (x+y=w119:fxp<+/-,64,36>)
              n103 = To Fixed-Point(fixed-point type=fxp<+/-,58,25> 0.0, number=w119) -> (fixed-point=w114:fxp<+/-,58,25>)
            }
            frame "Sawtooth Wave" {
              n104 = call "Saw Wave Generator.vi"("frequency (periods/tick)"=w131, "reset"=w132, "phase offset (periods)"=w130) -> ("saw out"=w129:i16)  [unwired: 12 in]
              n105 = Divide(x=w129, y=i16 32767) -> (x/y=w136:fxp<+/-,41,18>)
              n106 = Multiply(x=w136, y=w126) -> (x*y=w135:fxp<+/-,64,35>)
              n107 = Add(x=w135, y=w127) -> (x+y=w134:fxp<+/-,64,36>)
              n108 = To Fixed-Point(fixed-point type=fxp<+/-,58,25> 0.0, number=w134) -> (fixed-point=w128:fxp<+/-,58,25>)
            }
            frame "Square Wave" {
              w149 = fxp<+/-,32,16> 0.0 ("fixed-point type")
              n109 = call "Sine Wave Generator5"("frequency (periods/tick)"=w147, "reset"=w148, "phase offset (periods)"=w146) -> ("sine out"=w145:i16)  [unwired: 12 in]
              n110 = Divide(x=w145, y=i16 32767) -> (x/y=w169:fxp<+/-,41,18>)
              n111 = Greater?(x=w169, y=w149) -> (0:w156:bool)
              n112 = Less?(x=w169, y=w149) -> (x < y?=w155:bool)
              n113 = Equal?(x=w169, y=w149) -> (x = y?=w157:bool)
              n114 = Not(x=w156) -> (.not. x?=w153:bool)
              n115 = Not(x=w155) -> (.not. x?=w154:bool)
              n116 = Not(x=w157) -> (.not. x?=w152:bool)
              n117 = Compound Arithmetic op=AND(w156, w152, w154) -> (w158:bool)
              n118 = Compound Arithmetic op=AND(w153, w157, w154) -> (w151:bool)
              n119 = Compound Arithmetic op=AND(w153, w152, w155) -> (w150:bool)
              n120 = Select(t=fxp<+/-,2,2> 1.0 ("fixed-point type"), s=w158, f=fxp<+/-,2,2> 0.0 ("fixed-point type")) -> (s? t:f=w162:fxp<+/-,2,2>)
              n121 = Select(t=fxp<+/-,2,2> 0.0 ("fixed-point type"), s=w151, f=fxp<+/-,2,2> 0.0 ("fixed-point type")) -> (s? t:f=w161:fxp<+/-,2,2>)
              n122 = Add(x=w162, y=w161) -> (x+y=w160:fxp<+/-,3,3>)
              n123 = Select(t=fxp<+/-,2,2> -1.0 ("fixed-point type"), s=w150, f=fxp<+/-,2,2> 0.0 ("fixed-point type")) -> (s? t:f=w159:fxp<+/-,2,2>)
              n124 = Add(x=w160, y=w159) -> (x+y=w141:fxp<+/-,4,4>)
              n125 = Multiply(x=w141, y=w140) -> (x*y=w142:fxp<+/-,43,20>)
              n126 = Add(x=w142, y=w138) -> (x+y=w139:fxp<+/-,43,20>)
              n127 = To Fixed-Point(fixed-point type=fxp<+/-,58,25> 0.0, number=w139) -> (fixed-point=w143:fxp<+/-,58,25>)
            }
            frame "Filtered White Noise" {
              n128 = call "White Noise Generator3"("seed"=w183, "reset"=w181, "amplitude"=w182) -> ("white noise out"=w180:i16)  [unwired: 12 in]
              n129 = xnode "Butterworth Filter"("input data"=w180, "reset"=w181) -> ("output data"=w175:i16)  [unwired: 1 in]
              n130 = Divide(x=w175, y=i16 32767) -> (x/y=w178:fxp<+/-,41,18>)
              n131 = Multiply(x=w178, y=w173) -> (x*y=w177:fxp<+/-,64,35>)
              n132 = Add(x=w177, y=w172) -> (x+y=w176:fxp<+/-,64,36>)
              n133 = To Fixed-Point(fixed-point type=fxp<+/-,58,25> 0.0, number=w176) -> (fixed-point=w171:fxp<+/-,58,25>)
            }
          }
          "Z Stage Reference (nm)" <- w96
          n134 = local read "stop case"() -> (w95:bool)
        }
        n135 = while {
          shift-right: [w577] -> _
          shift-left: _ -> [w568]
          shift-right: [w576] -> _
          shift-left: _ -> [w567]
          shift-right: [w575] -> _
          shift-left: _ -> [w566]
          shift-right: [w574] -> _
          shift-left: _ -> [w565]
          shift-right: [w573] -> _
          shift-left: _ -> [w564]
          shift-right: [w572] -> _
          shift-left: _ -> [w563]
          shift-right: [w571] -> _
          shift-left: _ -> [w562]
          shift-right: [w570] -> _
          shift-left: _ -> [w561]
          shift-right: [w569] -> _
          shift-left: _ -> [w560]
          stop <- w589 stop-if-true
          w555 = fxp<+/-,20,5> 0.0 ("fixed-point type")
          n136 = local read "Sample X Stage Displacement (nm)"() -> (w551:fxp<+/-,58,25>)
          n137 = local read "Sample Y Stage Displacement (nm)"() -> (w548:fxp<+/-,58,25>)
          n138 = local read "Sample Z Stage Displacement (nm)"() -> (w545:fxp<+/-,58,25>)
          n139 = local read "Optics Z Stage Displacement (nm)"() -> (w544:fxp<+/-,58,25>)
          n140 = local read "Optics X Stage Displacement (nm)"() -> (w550:fxp<+/-,58,25>)
          n141 = local read "Optics Y Stage Displacement (nm)"() -> (w547:fxp<+/-,58,25>)
          n142 = case shown="\"FPGA Generated Reference\", Default" "Reference Signal Source" {
            tunnel: [w593 w596] -> w554
            tunnel: [w592 w595] -> w553
            tunnel: [w591 w594] -> w552
            frame "FPGA Generated Reference", Default {
              n143 = local read "X Stage Reference (nm)"() -> (w593:fxp<+/-,58,25>)
              n144 = local read "Y Stage Reference (nm)"() -> (w592:fxp<+/-,58,25>)
              n145 = local read "Z Stage Reference (nm)"() -> (w591:fxp<+/-,58,25>)
            }
            frame "External Reference" {
              n146 = local read "X Stage External Reference (nm)"() -> (w596:fxp<+/-,58,25>)
              n147 = local read "Y Stage External Reference (nm)"() -> (w595:fxp<+/-,58,25>)
              n148 = local read "Z Stage External Reference (nm)"() -> (w594:fxp<+/-,58,25>)
            }
          }
          n149 = call "Loop Timer3"("Count(uSec)"="Controller Time Period (uSec)") -> ()  [unwired: 1 out]
          n150 = case shown="\"Optics Stage Only\", Default" "Optics and or Sample Stage" {
            tunnel: w551 -> [_ w608]
            tunnel: w550 -> [w599 w607]
            tunnel: [w599 w606] -> w549
            tunnel: w548 -> [_ w605]
            tunnel: w547 -> [w598 w604]
            tunnel: [w598 w603] -> w546
            tunnel: w545 -> [_ w602]
            tunnel: w544 -> [w597 w601]
            tunnel: [w597 w600] -> w543
            frame "Optics Stage Only", Default {
            }
            frame "Optics and Sample Stage" {
              n151 = Subtract(x=w607, y=w608) -> (x-y=w606:fxp<+/-,59,26>)
              n152 = Subtract(x=w604, y=w605) -> (x-y=w603:fxp<+/-,59,26>)
              n153 = Subtract(x=w601, y=w602) -> (x-y=w600:fxp<+/-,59,26>)
            }
          }
          n154 = case shown="\"Closed Loop\"" "System Loop Type" {
            tunnel: w549 -> [_ w664]
            tunnel: w554 -> [w624 w665]
            tunnel: [w617 w638] -> w579
            tunnel: [w618 w663] -> w559
            tunnel: [_ w660] -> w577
            tunnel: [_ w659] -> w576
            tunnel: [_ w658] -> w575
            tunnel: [_ w657] -> w574
            tunnel: [_ w656] -> w573
            tunnel: [_ w655] -> w572
            tunnel: [_ w654] -> w571
            tunnel: [_ w653] -> w570
            tunnel: [_ w652] -> w569
            tunnel: w567 -> [_ w651]
            tunnel: w566 -> [_ w650]
            tunnel: w565 -> [_ w649]
            tunnel: w564 -> [_ w648]
            tunnel: w563 -> [_ w647]
            tunnel: w562 -> [_ w646]
            tunnel: w561 -> [_ w645]
            tunnel: w560 -> [_ w644]
            tunnel: w546 -> [_ w642]
            tunnel: w553 -> [w623 w643]
            tunnel: w552 -> [w622 w636]
            tunnel: w543 -> [_ w635]
            tunnel: [w616 w639] -> w578
            tunnel: w568 -> [_ w641]
            frame "Open Loop", Default {
              w615 = fxp<+/-,58,25> 0.0 ("fixed-point type")
              n155 = Multiply(x="X-Stage nm to V Scaling", y="X-Stage Scaling Direction") -> (x*y=w626:fxp<+/-,35,15>)
              n156 = Multiply(x="Y-Stage nm to V Scaling", y="Y-Stage Scaling Direction") -> (x*y=w612:fxp<+/-,35,15>)
              n157 = Multiply(x="Z-Stage nm to V Scaling", y="Z-Stage Scaling Direction") -> (x*y=w611:fxp<+/-,35,15>)
              n158 = Multiply(x=w624, y=w626) -> (x*y=w621:fxp<+/-,64,38>)
              n159 = Multiply(x=w623, y=w612) -> (x*y=w620:fxp<+/-,64,38>)
              n160 = Multiply(x=w622, y=w611) -> (x*y=w619:fxp<+/-,64,38>)
              n161 = To Fixed-Point(fixed-point type=w615, number=w621) -> (fixed-point=w618:fxp<+/-,58,25>)
              n162 = To Fixed-Point(fixed-point type=w615, number=w620) -> (fixed-point=w617:fxp<+/-,58,25>)
              n163 = To Fixed-Point(fixed-point type=w615, number=w619) -> (fixed-point=w616:fxp<+/-,58,25>)
            }
            frame "Closed Loop" {
              w631 = fxp<+/-,58,25> 0.0 ("fixed-point type")
              w632 = fxp<+/-,58,25> 0.0 ("fixed-point type")
              n164 = Subtract(x=w665, y=w664) -> (x-y=w669:fxp<+/-,60,27>)
              n165 = Subtract(x=w643, y=w642) -> (x-y=w668:fxp<+/-,60,27>)
              n166 = Subtract(x=w636, y=w635) -> (x-y=w637:fxp<+/-,60,27>)
              n167 = To Fixed-Point(fixed-point type=w631, number=w669) -> (fixed-point=w667:fxp<+/-,58,25>)
              n168 = To Fixed-Point(fixed-point type=w631, number=w668) -> (fixed-point=w666:fxp<+/-,58,25>)
              n169 = To Fixed-Point(fixed-point type=w631, number=w637) -> (fixed-point=w634:fxp<+/-,58,25>)
              n170 = for {
                N: 3 -> [_]
                shift-right: [w748] -> w630
                shift-left: _ -> [w746]
                shift-right: [w745] -> w629
                shift-left: _ -> [w743]
                tunnel: [w736] -> w660
                shift-right: [w735] -> _
                shift-left: _ -> [w731]
                tunnel: [w734] -> w659
                shift-right: [w733] -> _
                shift-left: _ -> [w729]
                tunnel: w641 -> [w726]
                tunnel: w651 -> [w725]
                tunnel: [w724] -> w657
                shift-right: [w723] -> _
                shift-left: _ -> [w716]
                tunnel: [w722] -> w656
                shift-right: [w721] -> _
                shift-left: _ -> [w715]
                tunnel: [w720] -> w654
                tunnel: [w719] -> w653
                shift-right: [w718] -> _
                shift-left: _ -> [w714]
                shift-right: [w717] -> _
                shift-left: _ -> [w703]
                tunnel: w649 -> [w713]
                tunnel: w648 -> [w712]
                tunnel: w646 -> [w711]
                tunnel: w645 -> [w710]
                tunnel: w667 -> [w702]
                tunnel: w666 -> [w699]
                shift-right: [w698] -> w628
                shift-left: _ -> [w695]
                tunnel: [w690] -> w658
                tunnel: [w689] -> w655
                tunnel: [w688] -> w652
                shift-right: [w687] -> _
                shift-left: _ -> [w683]
                shift-right: [w686] -> _
                shift-left: _ -> [w681]
                shift-right: [w685] -> _
                shift-left: _ -> [w679]
                tunnel: w650 -> [w678]
                tunnel: w644 -> [w677]
                tunnel: w647 -> [w676]
                tunnel: w634 -> [w672]
                i -> [w753]
                # "ez"
                # "ey"
                # "ex"
                n171 = Add(x=1, y=w753) -> (x+y=w671:i32)
                n172 = flat-sequence {
                  tunnel: [w796] -> w763
                  tunnel: [w795] -> w762
                  tunnel: [w794] -> w761
                  tunnel: [w793] -> w760
                  tunnel: [w792] -> w759
                  tunnel: [w791] -> w758
                  tunnel: [w790] -> w757
                  tunnel: [w789] -> w756
                  tunnel: w671 -> [w797]
                  tunnel: [w775] -> w755
                  tunnel: [w788] -> w747
                  tunnel: w746 -> [w788]
                  tunnel: [w787] -> w744
                  tunnel: w743 -> [w787]
                  tunnel: [w786] -> w732
                  tunnel: w731 -> [w786]
                  tunnel: [w766] -> w730
                  tunnel: w729 -> [w766]
                  tunnel: w726 -> [w777]
                  tunnel: w725 -> [w778]
                  tunnel: w716 -> [w785]
                  tunnel: w715 -> [w784]
                  tunnel: w714 -> [w783]
                  tunnel: w713 -> [w779]
                  tunnel: w712 -> [w780]
                  tunnel: w711 -> [w781]
                  tunnel: w710 -> [w782]
                  tunnel: w703 -> [w776]
                  tunnel: [w785] -> w709
                  tunnel: [w784] -> w708
                  tunnel: [w783] -> w707
                  tunnel: w702 -> [w765]
                  tunnel: [w776] -> w701
                  tunnel: w699 -> [w764]
                  tunnel: [w774] -> w696
                  tunnel: w695 -> [w774]
                  tunnel: [w773] -> w684
                  tunnel: w683 -> [w773]
                  tunnel: [w772] -> w682
                  tunnel: w681 -> [w772]
                  tunnel: [w771] -> w680
                  tunnel: w679 -> [w771]
                  tunnel: w678 -> [w768]
                  tunnel: w677 -> [w770]
                  tunnel: w676 -> [w769]
                  tunnel: w672 -> [w767]
                  tunnel: w763 -> [w849]
                  tunnel: w762 -> [w848]
                  tunnel: w761 -> [w847]
                  tunnel: w760 -> [w827]
                  tunnel: w759 -> [w828]
                  tunnel: w758 -> [w829]
                  tunnel: w757 -> [w830]
                  tunnel: w756 -> [w831]
                  tunnel: w755 -> [w836]
                  tunnel: [w834] -> w752
                  tunnel: [w834] -> w751
                  tunnel: [w825] -> w750
                  tunnel: [w826] -> w749
                  tunnel: w747 -> [w826]
                  tunnel: w744 -> [w825]
                  tunnel: [w835] -> w742
                  tunnel: [w835] -> w741
                  tunnel: [w833] -> w740
                  tunnel: [w833] -> w739
                  tunnel: [w832] -> w738
                  tunnel: [w832] -> w737
                  tunnel: w732 -> [w846]
                  tunnel: w730 -> [w845]
                  tunnel: [w846] -> w728
                  tunnel: [w845] -> w727
                  tunnel: w709 -> [w844]
                  tunnel: w708 -> [w843]
                  tunnel: w707 -> [w842]
                  tunnel: [w844] -> w706
                  tunnel: [w843] -> w705
                  tunnel: [w842] -> w704
                  tunnel: w701 -> [w841]
                  tunnel: [w841] -> w700
                  tunnel: [w834] -> w697
                  tunnel: w696 -> [w840]
                  tunnel: [w840] -> w694
                  tunnel: [w835] -> w693
                  tunnel: [w833] -> w692
                  tunnel: [w832] -> w691
                  tunnel: w684 -> [w839]
                  tunnel: w682 -> [w838]
                  tunnel: w680 -> [w837]
                  tunnel: [w839] -> w675
                  tunnel: [w838] -> w674
                  tunnel: [w837] -> w673
                  tunnel: w752 -> [w877]
                  tunnel: w751 -> [w932]
                  tunnel: w671 -> [w876]
                  tunnel: w750 -> [w931]
                  tunnel: w749 -> [w878]
                  tunnel: [w881] -> w748
                  tunnel: [w880] -> w745
                  tunnel: w742 -> [w918]
                  tunnel: w741 -> [w917]
                  tunnel: w740 -> [w916]
                  tunnel: w739 -> [w915]
                  tunnel: w738 -> [w914]
                  tunnel: w737 -> [w913]
                  tunnel: [w912] -> w736
                  tunnel: [w912] -> w735
                  tunnel: [w911] -> w734
                  tunnel: [w911] -> w733
                  tunnel: w728 -> [w910]
                  tunnel: w727 -> [w909]
                  tunnel: [w908] -> w724
                  tunnel: [w908] -> w723
                  tunnel: [w907] -> w722
                  tunnel: [w907] -> w721
                  tunnel: [w906] -> w720
                  tunnel: [w905] -> w719
                  tunnel: [w906] -> w718
                  tunnel: [w905] -> w717
                  tunnel: w706 -> [w904]
                  tunnel: w705 -> [w903]
                  tunnel: w704 -> [w902]
                  tunnel: w700 -> [w901]
                  tunnel: [w879] -> w698
                  tunnel: w697 -> [w898]
                  tunnel: w694 -> [w897]
                  tunnel: w693 -> [w890]
                  tunnel: w692 -> [w889]
                  tunnel: w691 -> [w888]
                  tunnel: [w887] -> w690
                  tunnel: [w886] -> w689
                  tunnel: [w885] -> w688
                  tunnel: [w887] -> w687
                  tunnel: [w886] -> w686
                  tunnel: [w885] -> w685
                  tunnel: w675 -> [w884]
                  tunnel: w674 -> [w883]
                  tunnel: w673 -> [w882]
                  frame #0 {
                    n173 = case shown="1, Default" w797 {
                      tunnel: ["sos gain SF Controller xx1" "sos gain SF Controller yy1" "sos gain SF Controller zz1"] -> w793
                      tunnel: ["-a01(2) xx1" "-a01(2) yy1" "-a01(2) zz1"] -> w792
                      tunnel: ["-a02(2) xx1" "-a02(2) yy1" "-a02(2) zz1"] -> w791
                      tunnel: ["b01(2) xx1" "b01(2) yy1" "b01(2) zz1"] -> w790
                      tunnel: ["b02(2) xx1" "b02(2) yy1" "b02(2) zz1"] -> w789
                      tunnel: [w798 w809 w823] -> w794
                      tunnel: [w804 w808 w822] -> w795
                      tunnel: [w805 w807 w821] -> w796
                      tunnel: w777 -> [w805 _ _]
                      tunnel: w778 -> [_ w807 _]
                      tunnel: w779 -> [w804 _ _]
                      tunnel: w780 -> [_ w808 _]
                      tunnel: w781 -> [w798 _ _]
                      tunnel: w782 -> [_ w809 _]
                      tunnel: [w806 w815 w824] -> w775
                      tunnel: w765 -> [w806 _ _]
                      tunnel: w764 -> [_ w815 _]
                      tunnel: w770 -> [_ _ w823]
                      tunnel: w769 -> [_ _ w822]
                      tunnel: w768 -> [_ _ w821]
                      tunnel: w767 -> [_ _ w824]
                      frame 1, Default {
                      }
                      frame 2 {
                      }
                      frame 3 {
                      }
                    }
                  }
                  frame #1 {
                    # "n_i"
                    # "m_i"
                    # "l_i"
                    # "u_i"
                    n174 = Multiply(x=w836, y=w827) -> (x*y=w850:fxp<+/-,64,34>)
                    n175 = To Fixed-Point(number=w850) -> (fixed-point=w851:fxp<+/-,58,25>)  [unwired: 1 in]
                    n176 = for {
                      tunnel: w828 -> [w867] mode=indexing
                      tunnel: w831 -> [w864] mode=indexing
                      shift-right: [w869] -> w834
                      shift-left: w851 -> [w868]
                      tunnel: w829 -> [w866] mode=indexing
                      tunnel: w830 -> [w865] mode=indexing
                      tunnel: [w856] -> w835 mode=indexing
                      tunnel: w849 -> [w862] mode=indexing
                      tunnel: [w859] -> w833 mode=indexing
                      tunnel: w848 -> [w852] mode=indexing
                      tunnel: [w852] -> w832 mode=indexing
                      tunnel: w847 -> [w860] mode=indexing
                      # "b_1"
                      # "b_2"
                      # "n_i-1"
                      # "-a_2"
                      # "-a_1"
                      # "m_i-1"
                      # "l_i-1"
                      # "e_i"
                      n177 = To Fixed-Point(number=w862) -> (fixed-point=w875:fxp<+/-,58,25>)  [unwired: 1 in]
                      n178 = Add(x=w868, y=w875) -> (x+y=w861:fxp<+/-,59,26>)
                      n179 = To Fixed-Point(number=w861) -> (fixed-point=w859:fxp<+/-,58,25>)  [unwired: 1 in]
                      n180 = Multiply(x=w859, y=w867) -> (x*y=w874:fxp<+/-,64,34>)
                      n181 = Multiply(x=w860, y=w864) -> (x*y=w873:fxp<+/-,64,34>)
                      n182 = Multiply(x=w852, y=w866) -> (x*y=w870:fxp<+/-,64,34>)
                      n183 = To Fixed-Point(number=w874) -> (fixed-point=w855:fxp<+/-,58,25>)  [unwired: 1 in]
                      n184 = To Fixed-Point(number=w870) -> (fixed-point=w854:fxp<+/-,58,25>)  [unwired: 1 in]
                      n185 = To Fixed-Point(number=w873) -> (fixed-point=w853:fxp<+/-,58,25>)  [unwired: 1 in]
                      n186 = Add(x=w855, y=w854) -> (x+y=w863:fxp<+/-,59,26>)
                      n187 = To Fixed-Point(number=w863) -> (fixed-point=w856:fxp<+/-,58,25>)  [unwired: 1 in]
                      n188 = Multiply(x=w852, y=w865) -> (x*y=w871:fxp<+/-,64,34>)
                      n189 = To Fixed-Point(number=w871) -> (fixed-point=w857:fxp<+/-,58,25>)  [unwired: 1 in]
                      n190 = Add(x=w857, y=w853) -> (x+y=w872:fxp<+/-,59,26>)
                      n191 = To Fixed-Point(number=w872) -> (fixed-point=w858:fxp<+/-,58,25>)  [unwired: 1 in]
                      n192 = Add(x=w859, y=w858) -> (x+y=w869:fxp<+/-,58,25>)
                    }
                  }
                  frame #2 {
                    n193 = Equal?(x=3, y=w876) -> (x = y?=w899:bool)
                    n194 = Equal?(x=2, y=w876) -> (x = y?=w933:bool)
                    n195 = Equal?(x=1, y=w876) -> (x = y?=w935:bool)
                    n196 = Equal?(x=2, y=w876) -> (x = y?=w923:bool)
                    n197 = Equal?(x=2, y=w876) -> (x = y?=w927:bool)
                    n198 = Equal?(x=3, y=w876) -> (x = y?=w895:bool)
                    n199 = Equal?(x=2, y=w876) -> (x = y?=w919:bool)
                    n200 = Equal?(x=1, y=w876) -> (x = y?=w929:bool)
                    n201 = Equal?(x=1, y=w876) -> (x = y?=w925:bool)
                    n202 = Equal?(x=3, y=w876) -> (x = y?=w893:bool)
                    n203 = Equal?(x=1, y=w876) -> (x = y?=w921:bool)
                    n204 = Equal?(x=3, y=w876) -> (x = y?=w891:bool)
                    n205 = Select(t=w898, s=w899, f=w897) -> (s? t:f=w879:fxp<+/-,58,25>)
                    "Kzz Output, Kzz*ez (V)" <- w879
                    n206 = Select(t=w932, s=w933, f=w931) -> (s? t:f=w880:fxp<+/-,58,25>)
                    "Kyy Output, Kyy*ey (V)" <- w880
                    n207 = Select(t=w877, s=w935, f=w878) -> (s? t:f=w881:fxp<+/-,58,25>)
                    "Kxx Output, Kxx*ex (V)" <- w881
                    n208 = Select(t=w915, s=w923, f=w903) -> (s? t:f=w907:fxp<+/-,58,25>[])
                    n209 = Select(t=w917, s=w927, f=w909) -> (s? t:f=w911:fxp<+/-,58,25>[])
                    n210 = Select(t=w890, s=w895, f=w884) -> (s? t:f=w887:fxp<+/-,58,25>[])
                    n211 = Select(t=w913, s=w919, f=w901) -> (s? t:f=w905:fxp<+/-,58,25>[])
                    n212 = Select(t=w918, s=w929, f=w910) -> (s? t:f=w912:fxp<+/-,58,25>[])
                    n213 = Select(t=w916, s=w925, f=w904) -> (s? t:f=w908:fxp<+/-,58,25>[])
                    n214 = Select(t=w889, s=w893, f=w883) -> (s? t:f=w886:fxp<+/-,58,25>[])
                    n215 = Select(t=w914, s=w921, f=w902) -> (s? t:f=w906:fxp<+/-,58,25>[])
                    n216 = Select(t=w888, s=w891, f=w882) -> (s? t:f=w885:fxp<+/-,58,25>[])
                  }
                }
              }
              n217 = Multiply(x=w628, y="Scaling mV to V") -> (x*y=w662:fxp<+/-,64,35>)
              n218 = Multiply(x=w630, y="Scaling mV to V") -> (x*y=w661:fxp<+/-,64,35>)
              n219 = Multiply(x=w629, y="Scaling mV to V") -> (x*y=w640:fxp<+/-,64,35>)
              n220 = To Fixed-Point(fixed-point type=w632, number=w661) -> (fixed-point=w663:fxp<+/-,58,25>)
              n221 = To Fixed-Point(fixed-point type=w632, number=w640) -> (fixed-point=w638:fxp<+/-,58,25>)
              n222 = To Fixed-Point(fixed-point type=w632, number=w662) -> (fixed-point=w639:fxp<+/-,58,25>)
            }
          }
          n223 = local read "stop case"() -> (w589:bool)
          n224 = To Fixed-Point(fixed-point type=w555, number=w559) -> (fixed-point=w558:fxp<+/-,20,5>)
          n225 = To Fixed-Point(fixed-point type=w555, number=w579) -> (fixed-point=w557:fxp<+/-,20,5>)
          n226 = To Fixed-Point(fixed-point type=w555, number=w578) -> (fixed-point=w556:fxp<+/-,20,5>)
          n227 = call "measure_loop_rate_FPGA.vi"() -> ("Loop Rate (Ticks)"=→"Measured Controller Time Period (Ticks)":u32)  [unwired: 11 in]
          n228 = In Range and Coerce(upper limit="Controller Output Upper Limit", x=w558, lower limit="Controller Output Lower Limit") -> (coerced(x)=→"PI X-Stage Input (V)":fxp<+/-,20,5>, In Range?=→"X-Stage Input In Range?":bool)
          n229 = In Range and Coerce(upper limit="Controller Output Upper Limit", x=w557, lower limit="Controller Output Lower Limit") -> (coerced(x)=→"PI Y-Stage Input (V)":fxp<+/-,20,5>, In Range?=→"Y-Stage Input In Range?":bool)
          n230 = In Range and Coerce(upper limit="Controller Output Upper Limit", x=w556, lower limit="Controller Output Lower Limit") -> (coerced(x)=→"PI Z-Stage Input (V)":fxp<+/-,20,5>, In Range?=→"Z-Stage Input In Range?":bool)
        }
        n231 = while {
          shift-right: [w351] -> _
          shift-left: i16 0 -> [w350]
          shift-right: [w349] -> _
          shift-left: i16 0 -> [w348]
          stop <- w361 stop-if-true
          n232 = local read "Fly Scan Running"() -> (w340:bool)
          n233 = case shown="\"Square Wave 1\"" "Trigger Wave Generator" {
            tunnel: [w377 w421 w443] -> w352
            tunnel: [w375 _ _] -> w351
            tunnel: w350 -> [w374 _ _]
            tunnel: [w368 _ _] -> w349
            tunnel: w348 -> [w367 _ _]
            tunnel: "DT Reset" -> [_ w427 w448]
            tunnel: "DT Frequency (periods/tick)" -> [_ w426 w447]
            tunnel: "DT Phase Offset (periods)" -> [_ w425 w446]
            tunnel: "DT Duty Cycle (periods)" -> [_ w424 _]
            tunnel: "DT Reference Amplitude (V)" -> [_ w423 w445]
            tunnel: "DT Reference DC Offset (V)" -> [_ w422 w444]
            tunnel: w340 -> [w362 w420 w442]
            frame "Custom Square Wave ", Default {
              n234 = local read "If True End Trigger High"() -> (w366:bool)
              n235 = local read "If True End Trigger Low"() -> (w365:bool)
              n236 = Not(x=w366) -> (.not. x?=w364:bool)
              n237 = Compound Arithmetic op=AND(w365, w364) -> (w363:bool)
              n238 = local read "Trigger Generation Time Period (uSec)"() -> (w373:u32)
              n239 = case shown="True" w363 {
                tunnel: [Detector_Trigger_Control."Trigger Low" Detector_Trigger_Control."Trigger High"] -> w376
                frame False {
                }
                frame True {
                }
              }
              n240 = case shown="True" w362 {
                tunnel: [fxp<+/-,20,5> 0.0 ("Trigger High Level (V)") w383] -> w377
                tunnel: w376 -> [_ w391]
                tunnel: [_ w390] -> w375
                tunnel: w374 -> [_ w389]
                tunnel: w373 -> [_ w388]
                tunnel: "Trigger High Period (usec)" -> [_ w387]
                tunnel: "Trigger Low Period (usec)" -> [_ w386]
                tunnel: "Trigger High Level (V)" -> [_ w385]
                tunnel: "Trigger Low Level (V)" -> [_ w384]
                tunnel: [_ w382] -> w368
                tunnel: w367 -> [_ w381]
                frame False {
                  n241 = local write "If True End Trigger High"(FALSE ("If True End Trigger High")) -> ()
                  n242 = local write "If True End Trigger Low"(TRUE ("If True End Trigger Low")) -> ()
                }
                frame True {
                  n243 = case shown="\"Trigger High\", Default" w391 {
                    tunnel: [w402 _] -> w390
                    tunnel: w389 -> [w401 _]
                    tunnel: w388 -> [w398 w412]
                    tunnel: w387 -> [w396 _]
                    tunnel: w386 -> [_ w410]
                    tunnel: w385 -> [w393 _]
                    tunnel: w384 -> [_ w405]
                    tunnel: [w393 w405] -> w383
                    tunnel: [_ w415] -> w382
                    tunnel: w381 -> [_ w414]
                    frame "Trigger High", Default {
                      n244 = Increment(x=w401) -> (x+1=w399:i16)
                      n245 = Multiply(x=w399, y=w398) -> (x*y=w397:u32)
                      n246 = Less Or Equal?(x=w397, y=w396) -> (x <= y?=w395:bool)
                      "Trigger Mid High" <- w395
                      n247 = Greater?(x=w397, y=w396) -> (0:w392:bool)
                      "If True End Trigger High" <- w392
                      n248 = case shown="True" w392 {
                        frame False {
                        }
                        frame True {
                          n249 = local write "If True End Trigger Low"(FALSE) -> ()
                        }
                      }
                      n250 = Select(t=w399, s=w395, f=i16 0) -> (s? t:f=w400:i16)
                      n251 = Select(t=i16 0, s=w392, f=w400) -> (s? t:f=w402:i16)
                    }
                    frame "Trigger Low" {
                      n252 = Increment(x=w414) -> (x+1=w413:i16)
                      n253 = Multiply(x=w413, y=w412) -> (x*y=w411:u32)
                      n254 = Less Or Equal?(x=w411, y=w410) -> (x <= y?=w409:bool)
                      n255 = Greater?(x=w411, y=w410) -> (0:w406:bool)
                      "If True End Trigger Low" <- w406
                      n256 = case shown="True" w406 {
                        frame False {
                        }
                        frame True {
                          n257 = local write "If True End Trigger High"(FALSE) -> ()
                        }
                      }
                      n258 = Select(t=w413, s=w409, f=i16 0) -> (s? t:f=w407:i16)
                      n259 = Select(t=i16 0, s=w406, f=w407) -> (s? t:f=w415:i16)
                    }
                  }
                }
              }
            }
            frame "Square Wave 1" {
              n260 = case shown="True" w420 {
                tunnel: w427 -> [_ w435]
                tunnel: w426 -> [_ w434]
                tunnel: w425 -> [_ w433]
                tunnel: w424 -> [_ w432]
                tunnel: w423 -> [_ w431]
                tunnel: w422 -> [_ w430]
                tunnel: [fxp<+/-,58,25> 0.0 ("fixed-point type") w429] -> w421
                frame False {
                }
                frame True {
                  n261 = call "Square Wave Generator"("frequency (periods/tick)"=w434, "reset"=w435, "phase offset (periods)"=w433, "duty cycle (periods)"=w432) -> ("square wave out"=w441:i16)  [unwired: 11 in]
                  n262 = Divide(x=w441, y=i16 32767) -> (x/y=w439:fxp<+/-,41,18>)
                  n263 = Multiply(x=w439, y=w431) -> (x*y=w438:fxp<+/-,64,35>)
                  n264 = Add(x=w438, y=w430) -> (x+y=w437:fxp<+/-,64,36>)
                  n265 = To Fixed-Point(fixed-point type=fxp<+/-,58,25> 0.0, number=w437) -> (fixed-point=w429:fxp<+/-,58,25>)
                }
              }
            }
            frame "Square Wave 2" {
              n266 = case shown="True" w442 {
                tunnel: w447 -> [_ w455]
                tunnel: w446 -> [_ w454]
                tunnel: w448 -> [_ w453]
                tunnel: w445 -> [_ w452]
                tunnel: w444 -> [_ w451]
                tunnel: [fxp<+/-,58,25> 0.0 ("fixed-point type") w450] -> w443
                frame False {
                }
                frame True {
                  w461 = fxp<+/-,32,16> 0.0 ("fixed-point type")
                  n267 = call "Sine Wave Generator3"("frequency (periods/tick)"=w455, "reset"=w453, "phase offset (periods)"=w454) -> ("sine out"=w460:i16)  [unwired: 12 in]
                  n268 = Divide(x=w460, y=i16 32767) -> (x/y=w481:fxp<+/-,41,18>)
                  n269 = Greater?(x=w481, y=w461) -> (0:w468:bool)
                  n270 = Equal?(x=w481, y=w461) -> (x = y?=w469:bool)
                  n271 = Less?(x=w481, y=w461) -> (x < y?=w467:bool)
                  n272 = Not(x=w468) -> (.not. x?=w465:bool)
                  n273 = Not(x=w469) -> (.not. x?=w464:bool)
                  n274 = Not(x=w467) -> (.not. x?=w466:bool)
                  n275 = Compound Arithmetic op=AND(w468, w464, w466) -> (w470:bool)
                  n276 = Compound Arithmetic op=AND(w465, w469, w466) -> (w463:bool)
                  n277 = Compound Arithmetic op=AND(w465, w464, w467) -> (w462:bool)
                  n278 = Select(t=fxp<+/-,2,2> 1.0 ("fixed-point type"), s=w470, f=fxp<+/-,2,2> 0.0 ("fixed-point type")) -> (s? t:f=w474:fxp<+/-,2,2>)
                  n279 = Select(t=fxp<+/-,2,2> 0.0 ("fixed-point type"), s=w463, f=fxp<+/-,2,2> 0.0 ("fixed-point type")) -> (s? t:f=w473:fxp<+/-,2,2>)
                  n280 = Select(t=fxp<+/-,2,2> -1.0 ("fixed-point type"), s=w462, f=fxp<+/-,2,2> 0.0 ("fixed-point type")) -> (s? t:f=w471:fxp<+/-,2,2>)
                  n281 = Add(x=w474, y=w473) -> (x+y=w472:fxp<+/-,3,3>)
                  n282 = Add(x=w472, y=w471) -> (x+y=w457:fxp<+/-,4,4>)
                  n283 = Multiply(x=w457, y=w452) -> (x*y=w458:fxp<+/-,43,20>)
                  n284 = Add(x=w458, y=w451) -> (x+y=w456:fxp<+/-,43,20>)
                  n285 = To Fixed-Point(fixed-point type=fxp<+/-,58,25> 0.0, number=w456) -> (fixed-point=w450:fxp<+/-,58,25>)
                }
              }
            }
          }
          n286 = call "measure_loop_rate_FPGA.vi"() -> ("Loop Rate (Ticks)"=→"Measured Trigger Gen Time Period (Ticks)":u32)  [unwired: 11 in]
          n287 = To Fixed-Point(fixed-point type=fxp<+/-,20,5> 0.0, number=w352) -> (fixed-point=w353:fxp<+/-,20,5>)
          n288 = In Range and Coerce(upper limit="Detector Trigger Upper Limit (V)", x=w353, lower limit="Detector Trigger Lower Limit (V)") -> (coerced(x)=→"Detector Trigger (V)":fxp<+/-,20,5>, In Range?=→"Detector Trigger In Range?":bool)
          n289 = call "Loop Timer7"("Count(uSec)"="Trigger Generation Time Period (uSec)") -> ()  [unwired: 1 out]
          n290 = local read "stop case"() -> (w361:bool)
        }
        n291 = while {
          tunnel: [w532] -> w68
          stop <- w538 stop-if-true
          n292 = local read "Detector Trigger (V)"() -> (w531:fxp<+/-,20,5>)
          n293 = local read "PI X-Stage Input (V)"() -> (w535:fxp<+/-,20,5>)
          n294 = local read "PI Y-Stage Input (V)"() -> (w534:fxp<+/-,20,5>)
          n295 = local read "PI Z-Stage Input (V)"() -> (w533:fxp<+/-,20,5>)
          n296 = xnode "FPGA I/O Node"("Mod8/AO0"=w535, "Mod8/AO1"=w534, "Mod8/AO2"=w533, "Mod8/AO3"=w531) -> ("error out"=w532:errorcluster)  [unwired: 5 in, 4 out]
          n297 = call "Loop Timer4"("Count(uSec)"="Controller Output Time Period (uSec)") -> ()  [unwired: 1 out]
          n298 = call "measure_loop_rate_FPGA.vi"() -> ("Loop Rate (Ticks)"=→"Measured Controller Output Time Period (Ticks)" →"Measured Detector Trigger Time Period (Ticks)":u32)  [unwired: 11 in]
          n299 = local read "stop case"() -> (w537:bool)
          n300 = Unbundle By Name(w532) -> ("status"=w536:bool)
          n301 = Or(x=w536, y=w537) -> (x .or. y?=w538:bool)
        }
        n302 = while {
          shift-right: [w200] -> _
          shift-left: _ -> [w195]
          shift-right: [w199] -> _
          shift-left: u32 0 ("f") -> [w197]
          shift-right: [w198] -> _
          shift-left: u32 0 -> [w196]
          stop <- w201 stop-if-true
          n303 = case shown="\"Custom Ramp Wave\"" "Y Reference Wave Selection" {
            tunnel: "Y Reference Amplitude (nm)" -> [w218 w222 _ w323]
            tunnel: "Y Reference DC Offset (nm)" -> [w217 w221 _ w322]
            tunnel: [w213 w220 w248 w319] -> w209
            tunnel: "Y Frequency (periods/tick)" -> [_ w231 _ _]
            tunnel: "Y Phase Offset (periods)" -> [_ w230 _ _]
            tunnel: "Y Reference Reset" -> [_ w229 _ w328]
            tunnel: "Y White Noise Seed" -> [_ _ _ w331]
            tunnel: "Y White Noise Amplitude" -> [_ _ _ w330]
            tunnel: [_ _ w246 _] -> w200
            tunnel: [_ _ w244 _] -> w199
            tunnel: [_ _ w243 _] -> w198
            tunnel: w197 -> [_ _ w242 _]
            tunnel: w196 -> [_ _ w241 _]
            tunnel: w195 -> [_ _ w239 _]
            tunnel: "Y Ramp Period (usec)" -> [_ _ w235 _]
            tunnel: "Y Ramp End (nm)" -> [_ _ w234 _]
            tunnel: "Y Ramp Start (nm)" -> [_ _ w233 _]
            frame "Constant", Default {
              n304 = Multiply(x=i16 1 ("y"), y=w218) -> (x*y=w216:fxp<+/-,56,33>)
              n305 = Add(x=w216, y=w217) -> (x+y=w215:fxp<+/-,56,33>)
              n306 = To Fixed-Point(fixed-point type=fxp<+/-,58,25> 0.0, number=w215) -> (fixed-point=w213:fxp<+/-,58,25>)
            }
            frame "Sine Wave" {
              n307 = call "Sine Wave Generator4"("frequency (periods/tick)"=w231, "reset"=w229, "phase offset (periods)"=w230) -> ("sine out"=w228:i16)  [unwired: 12 in]
              n308 = Divide(x=w228, y=i16 32767) -> (x/y=w226:fxp<+/-,41,18>)
              n309 = Multiply(x=w226, y=w222) -> (x*y=w225:fxp<+/-,64,35>)
              n310 = Add(x=w225, y=w221) -> (x+y=w224:fxp<+/-,64,36>)
              n311 = To Fixed-Point(fixed-point type=fxp<+/-,58,25> 0.0, number=w224) -> (fixed-point=w220:fxp<+/-,58,25>)
            }
            frame "Custom Ramp Wave" {
              n312 = Subtract(x=w233, y=w234) -> (x-y=w253:fxp<+/-,17,17>)
              n313 = Less?(x=w233, y=w234) -> (x < y?=w238:bool)
              n314 = Absolute Value(x=w253) -> (abs(x)=w252:fxp<+,16,16>)
              n315 = local read "Continue Run"() -> (w237:bool)
              n316 = Divide(x=w252, y=w235) -> (x/y=w254:fxp<+,48,16>)
              "Y Ramp Slope" <- w254
              n317 = local read "Start or middle"() -> (w250:bool)
              n318 = local read "Y Reference Time Period (uSec)"() -> (w240:u32)
              n319 = case shown="False" w238 {
                tunnel: [Control_Y_Up_Down_Ramp."Y Down Ramp" Control_Y_Up_Down_Ramp."Y Up Ramp"] -> w236
                frame False {
                }
                frame True {
                }
              }
              n320 = Compound Arithmetic op=OR("Fly Scan", w237) -> (w245:bool)
              "Fly Scan Running" <- w245
              n321 = Select(t=w239, s=w250, f=w233) -> (s? t:f=w251:fxp<+/-,58,25>)
              n322 = case shown="True" w245 {
                tunnel: w236 -> [_ w272]
                tunnel: w240 -> [_ w271]
                tunnel: ["Y Start Marker (nm)" w270] -> w249
                tunnel: w235 -> [_ w269]
                tunnel: w254 -> [_ w268]
                tunnel: w233 -> [_ w267]
                tunnel: w234 -> [_ w266]
                tunnel: [_ w265] -> w244
                tunnel: [_ w264] -> w243
                tunnel: w242 -> [_ w263]
                tunnel: w241 -> [_ w262]
                tunnel: [_ w261] -> w246
                tunnel: w251 -> [_ w260]
                frame False {
                  "Start or middle" <- FALSE ("Start or middle")
                  "Y scan done" <- TRUE
                }
                frame True {
                  n323 = case shown="\"Y Down Ramp\"" w272 {
                    tunnel: [w291 _] -> w265
                    tunnel: w263 -> [w290 _]
                    tunnel: w271 -> [w287 w308]
                    tunnel: w269 -> [w286 w304]
                    tunnel: w267 -> [w276 _]
                    tunnel: w266 -> [w280 w297]
                    tunnel: [_ w311] -> w264
                    tunnel: w262 -> [_ w310]
                    tunnel: w268 -> [w282 _]
                    tunnel: [w274 w293] -> w270
                    tunnel: [_ w293] -> w261
                    tunnel: w260 -> [_ w295]
                    frame "Y Up Ramp", Default {
                      n324 = Increment(x=w290) -> (x+1=w288:u32)
                      n325 = Multiply(x=w288, y=w287) -> (x*y=w283:u32)
                      n326 = Multiply(x=w283, y=w282) -> (x*y=w281:fxp<+,64,48>)
                      n327 = Less Or Equal?(x=w283, y=w286) -> (x <= y?=w285:bool)
                      "Ramp Mid Range" <- w285
                      n328 = Add(x=w281, y=w276) -> (x+y=w279:fxp<+/-,64,50>)
                      n329 = Greater?(x=w283, y=w286) -> (0:w275:bool)
                      "If True End Up Ramp" <- w275
                      n330 = Greater?(x=w279, y=w280) -> (0:w277:bool)
                      n331 = Select(t=w288, s=w285, f=i16 0) -> (s? t:f=w289:u32)
                      n332 = Select(t=w276, s=w277, f=w279) -> (s? t:f=w278:fxp<+/-,64,50>)
                      n333 = Select(t=i16 0, s=w275, f=w289) -> (s? t:f=w291:u32)
                      n334 = To Fixed-Point(fixed-point type=fxp<+/-,58,25> 0.0, number=w278) -> (fixed-point=w274:fxp<+/-,58,25>)
                    }
                    frame "Y Down Ramp" {
                      n335 = Increment(x=w310) -> (x+1=w309:u32)
                      n336 = local read "Y Ramp Drop"() -> (w301:bool)
                      n337 = Multiply(x=w309, y=w308) -> (x*y=w303:u32)
                      n338 = Less Or Equal?(x=w303, y=w304) -> (x <= y?=w307:bool)
                      n339 = Greater?(x=w303, y=w304) -> (0:w302:bool)
                      "If True End Y Down Ramp" <- w302
                      n340 = case shown="True" w301 {
                        tunnel: "Y Ramp Drop Size (nm)" -> [_ w316]
                        tunnel: [w313 w315] -> w299
                        tunnel: w295 -> [w313 w314]
                        frame False {
                        }
                        frame True {
                          n341 = Subtract(x=w314, y=w316) -> (x-y=w315:fxp<+/-,59,26>)
                        }
                      }
                      n342 = Select(t=w309, s=w307, f=u32 0) -> (s? t:f=w305:u32)
                      n343 = To Fixed-Point(fixed-point type=fxp<+/-,58,25> 0.0, number=w299) -> (fixed-point=w294:fxp<+/-,58,25>)
                      n344 = Less?(x=w294, y=w297) -> (x < y?=w296:bool)
                      n345 = case shown="True" w296 {
                        frame False {
                        }
                        frame True {
                          n346 = local write "Fly Scan Running"(FALSE ("Fly Scan Running")) -> ()
                          n347 = local write "Continue Run"(FALSE ("Start Scan")) -> ()
                        }
                      }
                      n348 = Select(t=u32 0, s=w302, f=w305) -> (s? t:f=w311:u32)
                      n349 = Select(t=w295, s=w296, f=w294) -> (s? t:f=w293:fxp<+/-,58,25>)
                    }
                  }
                }
              }
              n350 = To Fixed-Point(fixed-point type=fxp<+/-,58,25> 0.0, number=w249) -> (fixed-point=w248:fxp<+/-,58,25>)
            }
            frame "Filtered White Noise" {
              n351 = call "White Noise Generator2"("seed"=w331, "reset"=w328, "amplitude"=w330) -> ("white noise out"=w329:i16)  [unwired: 12 in]
              n352 = xnode "Butterworth Filter"("input data"=w329, "reset"=w328) -> ("output data"=w326:i16)  [unwired: 1 in]
              n353 = Divide(x=w326, y=i16 32767) -> (x/y=w325:fxp<+/-,41,18>)
              n354 = Multiply(x=w325, y=w323) -> (x*y=w324:fxp<+/-,64,35>)
              n355 = Add(x=w324, y=w322) -> (x+y=w321:fxp<+/-,64,36>)
              n356 = To Fixed-Point(fixed-point type=fxp<+/-,58,25> 0.0, number=w321) -> (fixed-point=w319:fxp<+/-,58,25>)
            }
          }
          "Y Stage Reference (nm)" <- w209
          n357 = call "measure_loop_rate_FPGA.vi"() -> ("Loop Rate (Ticks)"=→"Measured Y Reference Time Period (Ticks)":u32)  [unwired: 11 in]
          n358 = local read "stop case"() -> (w201:bool)
          n359 = call "Loop Timer9"("Count(uSec)"="Y Reference Time Period (uSec)") -> ()  [unwired: 1 out]
        }
        n360 = while {
          stop <- w529 stop-if-true
          w508 = fxp<+/-,58,25> 0.0 ("fixed-point type")
          n361 = local read "32 bit Count Sample  Y"() -> (w505:i32)
          n362 = local read "32 bit Count Sample  Z"() -> (w502:i32)
          n363 = local read "32 bit Count Sample X"() -> (w506:i32)
          n364 = local read "32 bit Count Optics  Y"() -> (w522:i32)
          n365 = local read "32 bit Count Optics  Z"() -> (w518:i32)
          n366 = local read "32 bit Count Optics X"() -> (w528:i32)
          n367 = Multiply(x=w528, y="Optics X Stage Resolution (nm)") -> (x*y=w525:fxp<+/-,64,35>)
          "Optics X Stage Displacement raw (nm)" <- w525
          n368 = Multiply(x=w506, y="Sample X Stage Resolution (nm)") -> (x*y=w514:fxp<+/-,64,35>)
          "Sample X Stage Displacement raw (nm)" <- w514
          n369 = Multiply(x=w522, y="Optics Y Stage Resolution (nm)") -> (x*y=w520:fxp<+/-,64,35>)
          "Optics Y Stage Displacement raw (nm)" <- w520
          n370 = Multiply(x=w505, y="Sample Y Stage Resolution (nm)") -> (x*y=w512:fxp<+/-,64,35>)
          "Sample Y Stage Displacement raw (nm)" <- w512
          n371 = Multiply(x=w518, y="Optics Z Stage Resolution (nm)") -> (x*y=w516:fxp<+/-,64,35>)
          "Optics Z Stage Displacement raw (nm)" <- w516
          n372 = Multiply(x=w502, y="Sample Z Stage Resolution (nm)") -> (x*y=w510:fxp<+/-,64,35>)
          "Sample Z Stage Displacement raw (nm)" <- w510
          n373 = call "Loop Timer5"("Count(uSec)"="Plant Output Time Period (uSec)") -> ()  [unwired: 1 out]
          n374 = call "measure_loop_rate_FPGA.vi"() -> ("Loop Rate (Ticks)"=→"Measured Plant Output Time Period (Ticks)":u32)  [unwired: 11 in]
          n375 = To Fixed-Point(fixed-point type=w508, number=w525) -> (fixed-point=→"Optics X Stage Displacement (nm)":fxp<+/-,58,25>)
          n376 = To Fixed-Point(fixed-point type=w508, number=w520) -> (fixed-point=→"Optics Y Stage Displacement (nm)":fxp<+/-,58,25>)
          n377 = To Fixed-Point(fixed-point type=w508, number=w516) -> (fixed-point=→"Optics Z Stage Displacement (nm)":fxp<+/-,58,25>)
          n378 = To Fixed-Point(fixed-point type=w508, number=w514) -> (fixed-point=→"Sample X Stage Displacement (nm)":fxp<+/-,58,25>)
          n379 = To Fixed-Point(fixed-point type=w508, number=w512) -> (fixed-point=→"Sample Y Stage Displacement (nm)":fxp<+/-,58,25>)
          n380 = To Fixed-Point(fixed-point type=w508, number=w510) -> (fixed-point=→"Sample Z Stage Displacement (nm)":fxp<+/-,58,25>)
          n381 = local read "stop case"() -> (w529:bool)
        }
        n382 = while {
          tunnel: [w485] -> w78
          stop <- w483 stop-if-true
          w487 = fxp<+/-,58,25> 0.0 ("fixed-point type")
          n383 = xnode "FPGA I/O Node"() -> ("error out"=w485:errorcluster, "Mod3/AI0"=w498:fxp<+/-,24,5>, "Mod3/AI1"=w489:fxp<+/-,24,5>, "Mod3/AI2"=w488:fxp<+/-,24,5>)  [unwired: 4 in, 3 out]
          "Mod 3 Input AI0 (V)" <- w498
          "Mod 8 Input AI1 (V)" <- w489
          "Mod 8 Input AI2 (V)" <- w488
          n384 = call "Loop Timer6"("Count(uSec)"="Analog Input Time Period (uSec)") -> ()  [unwired: 1 out]
          n385 = Multiply(x=w488, y="Mod 3 AI2 V to nm Scaling") -> (x*y=w491:fxp<+/-,64,23>)
          n386 = Multiply(x=w489, y="Mod 3 AI1 V to nm Scaling") -> (x*y=w494:fxp<+/-,64,23>)
          n387 = Multiply(x=w498, y="Mod 3 AI0 V to nm Scaling") -> (x*y=w500:fxp<+/-,64,23>)
          n388 = To Fixed-Point(fixed-point type=w487, number=w500) -> (fixed-point=→"X Stage External Reference (nm)":fxp<+/-,58,25>)
          n389 = To Fixed-Point(fixed-point type=w487, number=w494) -> (fixed-point=→"Y Stage External Reference (nm)":fxp<+/-,58,25>)
          n390 = To Fixed-Point(fixed-point type=w487, number=w491) -> (fixed-point=→"Z Stage External Reference (nm)":fxp<+/-,58,25>)
          n391 = call "measure_loop_rate_FPGA.vi"() -> ("Loop Rate (Ticks)"=→"Measured Analog Input Time Period (Ticks)":u32)  [unwired: 11 in]
          n392 = local read "stop case"() -> (w484:bool)
          n393 = Unbundle By Name(w485) -> ("status"=w486:bool)
          n394 = Or(x=w486, y=w484) -> (x .or. y?=w483:bool)
        }
        n395 = while {
          stop <- w83 stop-if-true
          n396 = local read "DT Frequency (periods/tick)"() -> (w87:fxp<+,32,0>)
          n397 = local read "DT Phase Offset (periods)"() -> (w86:fxp<+,32,0>)
          n398 = local read "DT Duty Cycle (periods)"() -> (w85:fxp<+,32,0>)
          n399 = local read "DT Reset"() -> (w84:bool)
          n400 = call "Square Wave Generator2"("frequency (periods/tick)"=w87, "reset"=w84, "phase offset (periods)"=w86, "duty cycle (periods)"=w85) -> ("square wave out"=w94:i16)  [unwired: 11 in]
          n401 = call "Loop Timer11"("Count(uSec)"="Data Trigger Time Period (uSec)") -> ()  [unwired: 1 out]
          n402 = call "measure_loop_rate_FPGA.vi"() -> ("Loop Rate (Ticks)"=→"Measured Data Trigger Time Period (Ticks)":u32)  [unwired: 11 in]
          n403 = Divide(x=w94, y=i16 32767) -> (x/y=w90:fxp<+/-,41,18>)
          n404 = To Fixed-Point(fixed-point type=fxp<+/-,58,25> 0.0, number=w90) -> (fixed-point=→"Trigger for Data":fxp<+/-,58,25>)
          n405 = local read "stop case"() -> (w83:bool)
        }
        n406 = while {
          tunnel: [w953] -> w79
          shift-right: [w946] -> _
          shift-left: _ -> [w945]
          shift-right: [w942] -> _
          shift-left: _ -> [w941]
          stop <- w951 stop-if-true
          n407 = local read "Trigger for Data"() -> (w942:fxp<+/-,58,25>)
          n408 = local read "Detector Trigger (V)"() -> (w946:fxp<+/-,20,5>)
          n409 = local read "Fly Scan Running"() -> (w943:bool)
          n410 = Greater?(x=w942, y=w941) -> (0:w940:bool)
          n411 = Greater?(x=w946, y=w945) -> (0:w944:bool)
          n412 = case shown="True" w943 {
            tunnel: [w957 w970] -> w954
            tunnel: [w958 w969] -> w947
            tunnel: w944 -> [_ w968]
            tunnel: w940 -> [w956 _]
            frame False {
              w965 = 5  # # of Data Strings
              n413 = case shown="True" w956 {
                tunnel: w965 -> [_ w966]
                tunnel: fxp<+/-,58,25> 0.0 ("fixed-point type") -> [_ w967]
                tunnel: [_ w967] -> w963
                tunnel: [_ w967] -> w961
                tunnel: [_ w967] -> w960
                tunnel: [_ w967] -> w959
                tunnel: [_ w967] -> w962
                tunnel: [_ w966] -> w957
                frame False {
                }
                frame True {
                }
              }
              "Number of Data Strings 2" <- w957
              n414 = Build Array "Build Array"(w963, w962, w961, w960, w959) -> (w958:fxp<+/-,58,25>[])
            }
            frame True {
              n415 = case shown="True" w968 {
                tunnel: [_ w977] -> w970
                tunnel: [_ w973] -> w969
                frame False {
                }
                frame True {
                  w978 = 5  # # of Data Strings
                  n416 = local read "Sample X Stage Displacement (nm)"() -> (w984:fxp<+/-,58,25>)
                  n417 = local read "Sample Y Stage Displacement (nm)"() -> (w983:fxp<+/-,58,25>)
                  n418 = local read "Sample Z Stage Displacement (nm)"() -> (w982:fxp<+/-,58,25>)
                  n419 = local read "Optics X Stage Displacement (nm)"() -> (w988:fxp<+/-,58,25>)
                  n420 = local read "Optics Y Stage Displacement (nm)"() -> (w987:fxp<+/-,58,25>)
                  n421 = local read "Optics Z Stage Displacement (nm)"() -> (w985:fxp<+/-,58,25>)
                  n422 = local read "X Stage External Reference (nm)"() -> (w976:fxp<+/-,58,25>)
                  n423 = local read "Y Stage External Reference (nm)"() -> (w975:fxp<+/-,58,25>)
                  n424 = local read "Z Stage External Reference (nm)"() -> (w974:fxp<+/-,58,25>)
                  n425 = local read "X Stage Reference (nm)"() -> (w996:fxp<+/-,58,25>)
                  n426 = local read "Y Stage Reference (nm)"() -> (w981:fxp<+/-,58,25>)
                  n427 = local read "Z Stage Reference (nm)"() -> (w980:fxp<+/-,58,25>)
                  n428 = local read "Detector Trigger (V)"() -> (w972:fxp<+/-,20,5>)
                  n429 = local read "PI X-Stage Input (V)"() -> (w995:fxp<+/-,20,5>)
                  n430 = local read "PI Y-Stage Input (V)"() -> (w994:fxp<+/-,20,5>)
                  n431 = local read "PI Z-Stage Input (V)"() -> (w993:fxp<+/-,20,5>)
                  n432 = case shown="\"Data Log 16\"" "Datalog Cases" {
                    tunnel: fxp<+/-,58,25> 0.0 ("fixed-point type") -> [w998 w1011 w1020 w1033 w1042 w1057 w1070 w1082 w1100 w1112 w1122 w1134 w1145 w1157 w1168 w1180]
                    tunnel: [w1007 w1018 w1030 w1041 w1054 w1067 w1077 w1094 w1104 w1118 w1127 w1142 w1154 w1165 w1176 w1188] -> w991
                    tunnel: w996 -> [w1008 _ _ _ w1047 _ _ _ _ _ _ _ _ _ _ w1184]
                    tunnel: w995 -> [w1004 _ _ _ w1046 _ _ _ _ w1119 _ _ w1149 _ _ _]
                    tunnel: w994 -> [_ w1017 _ _ _ w1061 _ _ _ _ w1132 _ _ w1160 _ _]
                    tunnel: w993 -> [_ _ w1027 _ _ _ w1074 _ _ _ _ w1143 _ _ w1171 _]
                    tunnel: [w1006 w1010 w1029 w1035 w1053 w1066 w1076 w1090 w1103 w1113 w1126 w1141 w1153 w1164 w1175 w1187] -> w990
                    tunnel: [w1005 w1019 w1028 w1040 w1052 w1065 w1075 w1086 w1102 w1114 w1125 w1140 w1152 w1163 w1174 w1186] -> w989
                    tunnel: w988 -> [w1001 _ _ w1037 w1049 _ _ w1097 _ w1117 w1131 w1138 w1148 _ _ w1182]
                    tunnel: w987 -> [_ w1013 _ w1036 _ w1060 _ w1093 _ w1116 w1130 w1137 _ w1159 _ w1181]
                    tunnel: fxp<+/-,40,17> 0.0 ("fixed-point type") -> [w1000 w1012 w1022 w1031 w1044 w1056 w1068 w1081 w1098 w1109 w1121 w1133 w1147 w1156 w1167 _]
                    tunnel: w985 -> [_ _ w1023 w1034 _ _ w1073 w1089 _ w1110 w1129 w1136 _ _ w1170 _]
                    tunnel: w984 -> [_ _ _ _ w1048 _ _ w1096 w1107 _ _ _ _ _ _ _]
                    tunnel: w983 -> [_ _ _ _ _ w1059 _ w1092 w1106 _ _ _ _ _ _ _]
                    tunnel: w982 -> [_ _ _ _ _ _ w1072 w1088 w1105 _ _ _ _ _ _ _]
                    tunnel: w981 -> [_ w1016 _ _ _ w1062 _ _ _ _ _ _ _ _ _ w1183]
                    tunnel: w980 -> [_ _ w1026 _ _ _ w1078 _ _ _ _ _ _ _ _ _]
                    tunnel: [w1003 w1015 w1025 w1039 w1051 w1064 w1071 w1085 w1101 w1115 w1124 w1139 w1151 w1162 w1173 w1185] -> w979
                    tunnel: w978 -> [w1002 w1014 w1024 w1038 w1050 w1063 w1079 w1084 w1108 w1120 w1128 w1144 w1155 w1166 w1177 w1189]
                    tunnel: [w1002 w1014 w1024 w1038 w1050 w1063 w1079 w1084 w1108 w1120 w1128 w1144 w1155 w1166 w1177 w1189] -> w977
                    tunnel: w976 -> [_ _ _ _ _ _ _ _ _ _ _ _ w1150 _ _ _]
                    tunnel: w975 -> [_ _ _ _ _ _ _ _ _ _ _ _ _ w1161 _ _]
                    tunnel: w974 -> [_ _ _ _ _ _ _ _ _ _ _ _ _ _ w1172 _]
                    tunnel: w972 -> [_ _ _ _ _ _ _ _ _ _ _ _ _ _ _ w1179]
                    tunnel: [w999 w1009 w1021 w1032 w1043 w1055 w1069 w1083 w1099 w1111 w1123 w1135 w1146 w1158 w1169 w1178] -> w971
                    frame "Data Log 1", Default {
                      n433 = To Fixed-Point(fixed-point type=w998, number=w1008) -> (fixed-point=w1007:fxp<+/-,58,25>)
                      n434 = To Fixed-Point(fixed-point type=w998, number=w1004) -> (fixed-point=w1006:fxp<+/-,58,25>)
                      n435 = To Fixed-Point(fixed-point type=w998, number=w1001) -> (fixed-point=w1005:fxp<+/-,58,25>)
                      n436 = To Fixed-Point(fixed-point type=w998, number=w1000) -> (fixed-point=w1003:fxp<+/-,58,25>)
                      n437 = To Fixed-Point(fixed-point type=w998, number=w1000) -> (fixed-point=w999:fxp<+/-,58,25>)
                    }
                    frame "Data Log 2" {
                      n438 = To Fixed-Point(fixed-point type=w1011, number=w1016) -> (fixed-point=w1018:fxp<+/-,58,25>)
                      n439 = To Fixed-Point(fixed-point type=w1011, number=w1017) -> (fixed-point=w1010:fxp<+/-,58,25>)
                      n440 = To Fixed-Point(fixed-point type=w1011, number=w1013) -> (fixed-point=w1019:fxp<+/-,58,25>)
                      n441 = To Fixed-Point(fixed-point type=w1011, number=w1012) -> (fixed-point=w1015:fxp<+/-,58,25>)
                      n442 = To Fixed-Point(fixed-point type=w1011, number=w1012) -> (fixed-point=w1009:fxp<+/-,58,25>)
                    }
                    frame "Data Log 3" {
                      n443 = To Fixed-Point(fixed-point type=w1020, number=w1026) -> (fixed-point=w1030:fxp<+/-,58,25>)
                      n444 = To Fixed-Point(fixed-point type=w1020, number=w1027) -> (fixed-point=w1029:fxp<+/-,58,25>)
                      n445 = To Fixed-Point(fixed-point type=w1020, number=w1023) -> (fixed-point=w1028:fxp<+/-,58,25>)
                      n446 = To Fixed-Point(fixed-point type=w1020, number=w1022) -> (fixed-point=w1025:fxp<+/-,58,25>)
                      n447 = To Fixed-Point(fixed-point type=w1020, number=w1022) -> (fixed-point=w1021:fxp<+/-,58,25>)
                    }
                    frame "Data Log 4" {
                      n448 = To Fixed-Point(fixed-point type=w1033, number=w1037) -> (fixed-point=w1041:fxp<+/-,58,25>)
                      n449 = To Fixed-Point(fixed-point type=w1033, number=w1036) -> (fixed-point=w1035:fxp<+/-,58,25>)
                      n450 = To Fixed-Point(fixed-point type=w1033, number=w1034) -> (fixed-point=w1040:fxp<+/-,58,25>)
                      n451 = To Fixed-Point(fixed-point type=w1033, number=w1031) -> (fixed-point=w1039:fxp<+/-,58,25>)
                      n452 = To Fixed-Point(fixed-point type=w1033, number=w1031) -> (fixed-point=w1032:fxp<+/-,58,25>)
                    }
                    frame "Data Log 5" {
                      n453 = To Fixed-Point(fixed-point type=w1042, number=w1047) -> (fixed-point=w1054:fxp<+/-,58,25>)
                      n454 = Subtract(x=w1049, y=w1048) -> (x-y=w1045:fxp<+/-,59,26>)
                      n455 = To Fixed-Point(fixed-point type=w1042, number=w1046) -> (fixed-point=w1053:fxp<+/-,58,25>)
                      n456 = To Fixed-Point(fixed-point type=w1042, number=w1045) -> (fixed-point=w1052:fxp<+/-,58,25>)
                      n457 = To Fixed-Point(fixed-point type=w1042, number=w1044) -> (fixed-point=w1051:fxp<+/-,58,25>)
                      n458 = To Fixed-Point(fixed-point type=w1042, number=w1044) -> (fixed-point=w1043:fxp<+/-,58,25>)
                    }
                    frame "Data Log 6" {
                      n459 = To Fixed-Point(fixed-point type=w1057, number=w1062) -> (fixed-point=w1067:fxp<+/-,58,25>)
                      n460 = To Fixed-Point(fixed-point type=w1057, number=w1061) -> (fixed-point=w1066:fxp<+/-,58,25>)
                      n461 = Subtract(x=w1060, y=w1059) -> (x-y=w1058:fxp<+/-,59,26>)
                      n462 = To Fixed-Point(fixed-point type=w1057, number=w1058) -> (fixed-point=w1065:fxp<+/-,58,25>)
                      n463 = To Fixed-Point(fixed-point type=w1057, number=w1056) -> (fixed-point=w1064:fxp<+/-,58,25>)
                      n464 = To Fixed-Point(fixed-point type=w1057, number=w1056) -> (fixed-point=w1055:fxp<+/-,58,25>)
                    }
                    frame "Data Log 7" {
                      n465 = To Fixed-Point(fixed-point type=w1070, number=w1078) -> (fixed-point=w1077:fxp<+/-,58,25>)
                      n466 = To Fixed-Point(fixed-point type=w1070, number=w1074) -> (fixed-point=w1076:fxp<+/-,58,25>)
                      n467 = Subtract(x=w1073, y=w1072) -> (x-y=w1080:fxp<+/-,59,26>)
                      n468 = To Fixed-Point(fixed-point type=w1070, number=w1080) -> (fixed-point=w1075:fxp<+/-,58,25>)
                      n469 = To Fixed-Point(fixed-point type=w1070, number=w1068) -> (fixed-point=w1071:fxp<+/-,58,25>)
                      n470 = To Fixed-Point(fixed-point type=w1070, number=w1068) -> (fixed-point=w1069:fxp<+/-,58,25>)
                    }
                    frame "Data Log 8" {
                      n471 = Subtract(x=w1097, y=w1096) -> (x-y=w1095:fxp<+/-,59,26>)
                      n472 = Subtract(x=w1093, y=w1092) -> (x-y=w1091:fxp<+/-,59,26>)
                      n473 = To Fixed-Point(fixed-point type=w1082, number=w1095) -> (fixed-point=w1094:fxp<+/-,58,25>)
                      n474 = Subtract(x=w1089, y=w1088) -> (x-y=w1087:fxp<+/-,59,26>)
                      n475 = To Fixed-Point(fixed-point type=w1082, number=w1091) -> (fixed-point=w1090:fxp<+/-,58,25>)
                      n476 = To Fixed-Point(fixed-point type=w1082, number=w1087) -> (fixed-point=w1086:fxp<+/-,58,25>)
                      n477 = To Fixed-Point(fixed-point type=w1082, number=w1081) -> (fixed-point=w1085:fxp<+/-,58,25>)
                      n478 = To Fixed-Point(fixed-point type=w1082, number=w1081) -> (fixed-point=w1083:fxp<+/-,58,25>)
                    }
                    frame "Data Log 9" {
                      n479 = To Fixed-Point(fixed-point type=w1100, number=w1107) -> (fixed-point=w1104:fxp<+/-,58,25>)
                      n480 = To Fixed-Point(fixed-point type=w1100, number=w1106) -> (fixed-point=w1103:fxp<+/-,58,25>)
                      n481 = To Fixed-Point(fixed-point type=w1100, number=w1105) -> (fixed-point=w1102:fxp<+/-,58,25>)
                      n482 = To Fixed-Point(fixed-point type=w1100, number=w1098) -> (fixed-point=w1101:fxp<+/-,58,25>)
                      n483 = To Fixed-Point(fixed-point type=w1100, number=w1098) -> (fixed-point=w1099:fxp<+/-,58,25>)
                    }
                    frame "Data Log 10" {
                      n484 = To Fixed-Point(fixed-point type=w1112, number=w1119) -> (fixed-point=w1118:fxp<+/-,58,25>)
                      n485 = To Fixed-Point(fixed-point type=w1112, number=w1117) -> (fixed-point=w1113:fxp<+/-,58,25>)
                      n486 = To Fixed-Point(fixed-point type=w1112, number=w1116) -> (fixed-point=w1114:fxp<+/-,58,25>)
                      n487 = To Fixed-Point(fixed-point type=w1112, number=w1110) -> (fixed-point=w1115:fxp<+/-,58,25>)
                      n488 = To Fixed-Point(fixed-point type=w1112, number=w1109) -> (fixed-point=w1111:fxp<+/-,58,25>)
                    }
                    frame "Data Log 11" {
                      n489 = To Fixed-Point(fixed-point type=w1122, number=w1132) -> (fixed-point=w1127:fxp<+/-,58,25>)
                      n490 = To Fixed-Point(fixed-point type=w1122, number=w1131) -> (fixed-point=w1126:fxp<+/-,58,25>)
                      n491 = To Fixed-Point(fixed-point type=w1122, number=w1130) -> (fixed-point=w1125:fxp<+/-,58,25>)
                      n492 = To Fixed-Point(fixed-point type=w1122, number=w1129) -> (fixed-point=w1124:fxp<+/-,58,25>)
                      n493 = To Fixed-Point(fixed-point type=w1122, number=w1121) -> (fixed-point=w1123:fxp<+/-,58,25>)
                    }
                    frame "Data Log 12" {
                      n494 = To Fixed-Point(fixed-point type=w1134, number=w1143) -> (fixed-point=w1142:fxp<+/-,58,25>)
                      n495 = To Fixed-Point(fixed-point type=w1134, number=w1138) -> (fixed-point=w1141:fxp<+/-,58,25>)
                      n496 = To Fixed-Point(fixed-point type=w1134, number=w1137) -> (fixed-point=w1140:fxp<+/-,58,25>)
                      n497 = To Fixed-Point(fixed-point type=w1134, number=w1136) -> (fixed-point=w1139:fxp<+/-,58,25>)
                      n498 = To Fixed-Point(fixed-point type=w1134, number=w1133) -> (fixed-point=w1135:fxp<+/-,58,25>)
                    }
                    frame "Data Log 13" {
                      n499 = To Fixed-Point(fixed-point type=w1145, number=w1150) -> (fixed-point=w1154:fxp<+/-,58,25>)
                      n500 = To Fixed-Point(fixed-point type=w1145, number=w1149) -> (fixed-point=w1153:fxp<+/-,58,25>)
                      n501 = To Fixed-Point(fixed-point type=w1145, number=w1148) -> (fixed-point=w1152:fxp<+/-,58,25>)
                      n502 = To Fixed-Point(fixed-point type=w1145, number=w1147) -> (fixed-point=w1151:fxp<+/-,58,25>)
                      n503 = To Fixed-Point(fixed-point type=w1145, number=w1147) -> (fixed-point=w1146:fxp<+/-,58,25>)
                    }
                    frame "Data Log 14" {
                      n504 = To Fixed-Point(fixed-point type=w1157, number=w1161) -> (fixed-point=w1165:fxp<+/-,58,25>)
                      n505 = To Fixed-Point(fixed-point type=w1157, number=w1160) -> (fixed-point=w1164:fxp<+/-,58,25>)
                      n506 = To Fixed-Point(fixed-point type=w1157, number=w1159) -> (fixed-point=w1163:fxp<+/-,58,25>)
                      n507 = To Fixed-Point(fixed-point type=w1157, number=w1156) -> (fixed-point=w1162:fxp<+/-,58,25>)
                      n508 = To Fixed-Point(fixed-point type=w1157, number=w1156) -> (fixed-point=w1158:fxp<+/-,58,25>)
                    }
                    frame "Data Log 15" {
                      n509 = To Fixed-Point(fixed-point type=w1168, number=w1172) -> (fixed-point=w1176:fxp<+/-,58,25>)
                      n510 = To Fixed-Point(fixed-point type=w1168, number=w1171) -> (fixed-point=w1175:fxp<+/-,58,25>)
                      n511 = To Fixed-Point(fixed-point type=w1168, number=w1170) -> (fixed-point=w1174:fxp<+/-,58,25>)
                      n512 = To Fixed-Point(fixed-point type=w1168, number=w1167) -> (fixed-point=w1173:fxp<+/-,58,25>)
                      n513 = To Fixed-Point(fixed-point type=w1168, number=w1167) -> (fixed-point=w1169:fxp<+/-,58,25>)
                    }
                    frame "Data Log 16" {
                      n514 = To Fixed-Point(fixed-point type=w1180, number=w1184) -> (fixed-point=w1188:fxp<+/-,58,25>)
                      n515 = To Fixed-Point(fixed-point type=w1180, number=w1183) -> (fixed-point=w1187:fxp<+/-,58,25>)
                      n516 = To Fixed-Point(fixed-point type=w1180, number=w1182) -> (fixed-point=w1186:fxp<+/-,58,25>)
                      n517 = To Fixed-Point(fixed-point type=w1180, number=w1181) -> (fixed-point=w1185:fxp<+/-,58,25>)
                      n518 = To Fixed-Point(fixed-point type=w1180, number=w1179) -> (fixed-point=w1178:fxp<+/-,58,25>)
                    }
                  }
                  "Number of Data Strings" <- w977
                  n519 = Build Array "Build Array"(w991, w990, w989, w979, w971) -> (w973:fxp<+/-,58,25>[])
                }
              }
            }
          }
          n520 = call "Loop Timer2"("Count(uSec)"="Datalog Time Period (uSec)") -> ()  [unwired: 1 out]
          n521 = for {
            N: w954 -> [_]
            tunnel: w947 -> [w1197] mode=indexing
            shift-right: [w1195] -> w953
            shift-left: _ -> [w1194]
            shift-right: [w1191] -> w948
            shift-left: _ -> [w1192]
            n522 = xnode "FIFO"("Element"=w1197, "Timeout"="Timeout FPGA FIFO1", "error in (no error)"=w1194) -> ("Timed Out?"=w1193:bool, "error out"=w1195:errorcluster)  [unwired: 1 in, 1 out]
            "FIFO Timed Out?" <- w1193
            n523 = Or(x=w1193, y=w1192) -> (x .or. y?=w1191:bool)
          }
          "FIFO Timed Out" <- w948
          n524 = call "measure_loop_rate_FPGA.vi"() -> ("Loop Rate (Ticks)"=→"Measured Datalog Time Period (Ticks)":u32)  [unwired: 11 in]
          n525 = local read "stop case"() -> (w949:bool)
          n526 = local read "Y scan done"() -> (w939:bool)
          n527 = local read "X scan done"() -> (w938:bool)
          n528 = Unbundle By Name "Unbundle By Name"(w953) -> ("Status?"=w952:bool)
          n529 = And(x=w939, y=w938) -> (x .and. y?=w937:bool)
          "Fly scan completed" <- w937
          n530 = Compound Arithmetic op=OR(w952, w948, w949, w937) -> (w951:bool)
          n531 = case shown="True" w951 {
            selector: w951 -> [_ w1190]
            frame False {
            }
            frame True {
              n532 = local write "stop case"(w1190) -> ()
            }
          }
        }
        n533 = Merge Errors(w68, w78, w79) -> (w69:errorcluster)
        "Run Loop error" <- w69
        n534 = case shown="No Error" w69 {
          tunnel: [FPGA_states."End Run" FPGA_states."Wait"] -> w70
          frame No Error {
          }
          frame Error {
            n535 = local write "stop case"(TRUE) -> ()
          }
        }
      }
      frame "End Run" {
        n536 = xnode "FPGA I/O Node"("Mod3/Stop"=TRUE ("I/O Item")) -> ("error out"=w1343:errorcluster)  [unwired: 2 in, 1 out]
        "End Run Error" <- w1343
      }
      frame "Shutdown" {
        n537 = xnode "FPGA I/O Node"("error in"=w1348, "System Reset"=TRUE) -> ("error out"=w1347:errorcluster)  [unwired: 1 in, 1 out]
        "Shutdown error" <- w1347
      }
    }
    "FPGA state" <- w38
  }
  n538 = node-c288(refnum<k21> "40 MHz Onboard Clock" ("Source Name"), w1) -> (w6:T13)
  n539 = timed-loop {
    timing: w6 -> [_]
    timing-out: [_] -> w5
    shift-right: [w1382] -> _
    shift-left: _ -> [w1384]
    shift-right: [w1381] -> _
    shift-left: _ -> [w1383]
    shift-right: [w1403] -> _
    shift-left: w4 -> [w1400]
    shift-right: [w1402] -> _
    shift-left: u32 0 ("Tick Count(Ticks)") -> [w1401]
    shift-right: [w1373] -> _
    shift-left: _ -> [w1372]
    shift-right: [w1374] -> _
    shift-left: _ -> [w1371]
    shift-right: [w1396] -> _
    shift-left: w4 -> [w1395]
    shift-right: [w1361] -> _
    shift-left: _ -> [w1362]
    shift-right: [w1360] -> _
    shift-left: _ -> [w1363]
    shift-right: [w1390] -> _
    shift-left: w4 -> [w1389]
    shift-right: [w1379] -> _
    shift-left: _ -> [w1377]
    shift-right: [w1378] -> _
    shift-left: _ -> [w1376]
    shift-right: [w1399] -> _
    shift-left: w4 -> [w1398]
    shift-right: [w1366] -> _
    shift-left: _ -> [w1367]
    shift-right: [w1365] -> _
    shift-left: _ -> [w1368]
    shift-right: [w1393] -> _
    shift-left: w4 -> [w1392]
    shift-right: [w1356] -> _
    shift-left: _ -> [w1358]
    shift-right: [w1357] -> _
    shift-left: _ -> [w1359]
    shift-right: [w1388] -> _
    shift-left: w4 -> [w1386]
    shift-right: [w1353] -> _
    shift-left: _ -> [w1352]
    stop <- w1351 stop-if-true
    # "Tracks interferometer data"
    n540 = xnode "FPGA I/O Node"("error in"=w1352) -> ("error out"=w1375:errorcluster, "Mod4/DIO2"=w1379:bool, "Mod4/DIO3"=w1378:bool)  [unwired: 2 in, 2 out]
    "Mod4/DIO2" <- w1379
    "Mod4/DIO3" <- w1378
    n541 = xnode "FPGA I/O Node"("error in"=w1352) -> ("error out"=w1369:errorcluster, "Mod5/DIO2"=w1366:bool, "Mod5/DIO3"=w1365:bool)  [unwired: 2 in, 2 out]
    "Mod5/DIO2" <- w1366
    "Mod5/DIO3" <- w1365
    n542 = xnode "FPGA I/O Node"("error in"=w1352) -> ("error out"=w1355:errorcluster, "Mod6/DIO0"=w1361:bool, "Mod6/DIO1"=w1360:bool)  [unwired: 2 in, 2 out]
    "Mod6/DIO0" <- w1361
    "Mod6/DIO1" <- w1360
    n543 = xnode "FPGA I/O Node"("error in"=w1352) -> ("error out"=w1370:errorcluster, "Mod5/DIO0"=w1373:bool, "Mod5/DIO1"=w1374:bool)  [unwired: 2 in, 2 out]
    "Mod5/DIO0" <- w1373
    "Mod5/DIO1" <- w1374
    n544 = xnode ("FPGA I/O Node")("error in"=w1352) -> ("error out"=w1380:errorcluster, "Mod4/DIO0"=w1382:bool, "Mod4/DIO1"=w1381:bool)  [unwired: 2 in, 2 out]
    "Mod4/DIO0" <- w1382
    "Mod4/DIO1" <- w1381
    n545 = xnode "FPGA I/O Node"("error in"=w1352) -> ("error out"=w1354:errorcluster, "Mod6/DIO2"=w1356:bool, "Mod6/DIO3"=w1357:bool)  [unwired: 2 in, 2 out]
    "Mod6/DIO2" <- w1356
    "Mod6/DIO3" <- w1357
    n546 = call "Tick Count"() -> ("Tick Count(Ticks)"=w1402:u32)
    n547 = Subtract(x=w1402, y=w1401) -> (x-y=→"Measured Counter Time Period (Ticks)":u32)
    n548 = Merge Errors(w1380, w1375, w1370, w1369, w1355, w1354) -> (w1353:errorcluster)
    "Interferometer Loop Error" <- w1353
    n549 = call "Quadrature.vi"("Reset Counter"="Reset Optics X", "Quad A"=w1382, "ticks in"=w1400, "Last Quad B"=w1383, "Last Quad A"=w1384, "Quad B"=w1381) -> ("ticks out"=w1403:i32)  [unwired: 5 in]
    "32 bit Count Optics X" <- w1403
    n550 = call "Quadrature.vi"("Reset Counter"="Reset Sample X", "Quad A"=w1379, "ticks in"=w1398, "Last Quad B"=w1376, "Last Quad A"=w1377, "Quad B"=w1378) -> ("ticks out"=w1399:i32)  [unwired: 5 in]
    "32 bit Count Sample X" <- w1399
    n551 = call "Quadrature.vi"("Reset Counter"="Reset Optics Y", "Quad A"=w1373, "ticks in"=w1395, "Last Quad B"=w1371, "Last Quad A"=w1372, "Quad B"=w1374) -> ("ticks out"=w1396:i32)  [unwired: 5 in]
    "32 bit Count Optics  Y" <- w1396
    n552 = call "Quadrature.vi"("Reset Counter"="Reset Sample Y", "Quad A"=w1366, "ticks in"=w1392, "Last Quad B"=w1368, "Last Quad A"=w1367, "Quad B"=w1365) -> ("ticks out"=w1393:i32)  [unwired: 5 in]
    "32 bit Count Sample  Y" <- w1393
    n553 = call "Quadrature.vi"("Reset Counter"="Reset Optics Z", "Quad A"=w1361, "ticks in"=w1389, "Last Quad B"=w1363, "Last Quad A"=w1362, "Quad B"=w1360) -> ("ticks out"=w1390:i32)  [unwired: 5 in]
    "32 bit Count Optics  Z" <- w1390
    n554 = call "Quadrature.vi"("Reset Counter"="Reset Sample Z", "Quad A"=w1356, "ticks in"=w1386, "Last Quad B"=w1359, "Last Quad A"=w1358, "Quad B"=w1357) -> ("ticks out"=w1388:i32)  [unwired: 5 in]
    "32 bit Count Sample  Z" <- w1388
    n555 = Unbundle By Name(w1353) -> ("status"=w1351:bool)
  }
  n556 = node-c288(w5) -> ()  [unwired: 1 out]
